vi "XAVIER AUTO.vi"(6 "stop?":bool, 7 "Vision?":bool, 9 "Angle(degrees)":dbl, 10 "Cluster":cluster{"DriveRef":T1}, 11 "Auto Choice":T9(ring)) -> (3 "End?":bool)   [LabVIEW 2015]
uses:
  Robot Global Data.vi
  <vilib>/Rock Robotics/WPI/CAN/Jaguar/SubVIs/WPI_CANJaguar_ControlMode.ctl
  <vilib>/Rock Robotics/WPI/CAN/TalonSRX/WPI_CANTalonSRX_APIControlMode.ctl
  <vilib>/Rock Robotics/SystemInterfaces/DIO/FPGA_DIOPWMChannel.ctl
  <vilib>/Rock Robotics/WPI/PWM/WPI_PWMDeadband.ctl
  <vilib>/Rock Robotics/WPI/MotorControl/WPI_MotorControlType.ctl
  <vilib>/Rock Robotics/WPI/MotorControl/WPI_MotorControlDeviceRef.ctl
  <vilib>/Rock Robotics/WPI/RobotDrive/WPI_RobotDriveDevRef.ctl
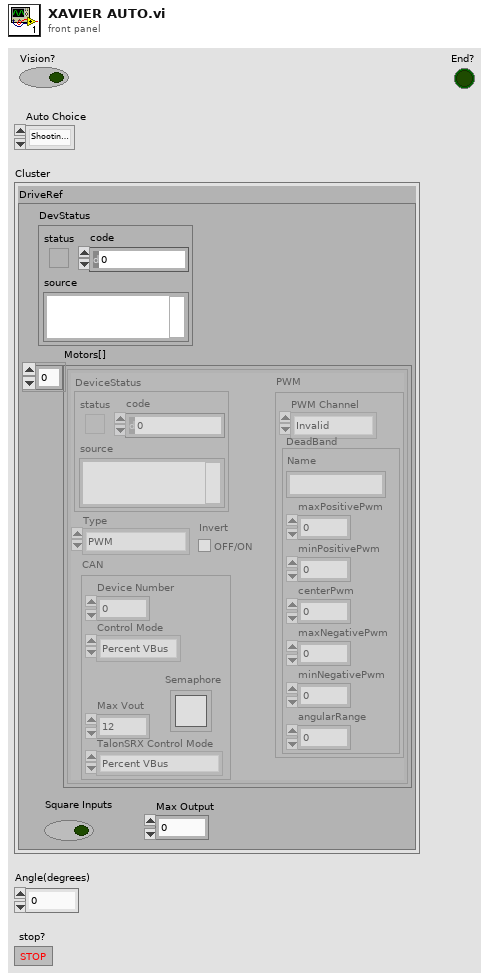
[diagram p1: front panel]
types:
  T1 = typedef "WPI_RobotDriveDevRef.ctl" = cluster{"DevStatus":errorcluster, "Motors[]":T2[], "Square Inputs":bool, "Max Output":dbl}
  T2 = typedef "WPI_MotorControlDeviceRef.ctl" = cluster{"DeviceStatus":errorcluster, "Type":T3, "PWM":cluster{"PWM Channel":T4, "DeadBand":T5}, "CAN":cluster{"Device Number":u8, "Control Mode":T6, "Semaphore":T7, "Max Vout":dbl, "TalonSRX Control Mode":T8}, "Invert":bool}
  T3 = typedef "WPI_MotorControlType.ctl" = enum16{"PWM", "CAN", "CANTalonSRX"}
  T4 = typedef "FPGA_DIOPWMChannel.ctl" = enum8{"PWM 0", "PWM 1", "PWM 2", "PWM 3", "PWM 4", "PWM 5", "PWM 6", "PWM 7", "PWM 8", "PWM 9", "PWM MXP 0", "PWM MXP 1", "PWM MXP 2", "PWM MXP 3", "PWM MXP 4", "PWM MXP 5", "PWM MXP 6", "PWM MXP 7", "PWM MXP 8", "PWM MXP 9", "Invalid"}
  T5 = typedef "WPI_PWMDeadband.ctl" = cluster{"Name":string, "maxPositivePwm":i32, "minPositivePwm":i32, "centerPwm":i32, "maxNegativePwm":i32, "minNegativePwm":i32, "angularRange":u16}
  T6 = typedef "WPI_CANJaguar_ControlMode.ctl" = enum8{"Percent VBus", "Current", "Speed", "Position", "Voltage"}
  T7 = typedef "Semaphore RefNum" = refnum<k1>
  T8 = typedef "WPI_CANTalonSRX_APIControlMode.ctl" = enum8{"Percent VBus", "Speed", "Position", "Slave", "Unchanged / Invalid", "Voltage Compensation", "Current", "Motion Profile"}
  T9 = enum16{"Shooting (Testing Only)", "Low Bar/Pos 2/Pos 3 (full)", "Low Bar/Pos 2/Pos 3 (no turn back)", "Low Bar/Pos 2/Pos 3 (move and turn test)", "Position 4", "Position 5", "Move Arms Down/Up Test", "Move Forward through Defense", "Turn Until Vision Test"}
  T10 = enum16{"Start", "Turn (No Vision)", "Turn (Vision)", "Shoot", "Turn Back", "Move Back", "End"}
  T11 = cluster{"y":dbl, "Distance":dbl, "Angle":dbl, "x":dbl}
  T12 = typedef "WPI_CANTalonSRX_GlobalStatus.ctl" = cluster{"Applied Throttle":dbl, "Module Enabled":bool, "CAN Error":errorcluster, "Closed Loop Error":dbl, "Forward Limit Switch Closed":bool, "Reverse Limit Switch Closed":bool, "Sensor Position":dbl, "Sensor Velocity":dbl, "Current":dbl, "Sticky Fault - Over Temp":bool, "Sticky Fault - Under Voltage":bool, "Sticky Fault - Forward Limit":bool, "Sticky Fault - Reverse Limit":bool, "Sticky Fault - Forward Soft Limit":bool, "Sticky Fault - Reverse Soft Limit":bool, "Brake is Enabled":bool, "Encoder Position":dbl, "Encoder Velocity":dbl, "Encoder Index Count":dbl, "Encoder A Pin State":bool, "Encoder B Pin State":bool, "Encoder Index Pin State":bool, "Analog In":dbl, "Analog In Velocity":dbl, "Temperature (C)":dbl, "Battery Voltage":dbl, "Control 5 Is Supported":bool, "Current Profile Slot Select":dbl, "Pos Div 8":bool, "Vel Div 4":bool, "Pulse Width Position":i32, "Pulse Width Velocity":i32, "Pulse Width Rise To Rise (us)":i32, "Pulse Width Rise To Fall (us)":i32, "Mot Prof Active Is Under Run":bool, "Mot Prof Active Has Under Run":bool, "Mot Prof Active Is Last":bool, "Mot Prof Active Velocity Only":bool, "Mot Prof Active Is Valid":bool, "Mot Prof Buffer Is Full":bool, "Mot Prof Active Profile Slot Select":i32, "Mot Prof NextID":i32, "Mot Prof Count":i32, "Mot Prof Active Velocity":dbl, "Mot Prof Active Position":dbl, "Mot Prof Output Enable":i32}
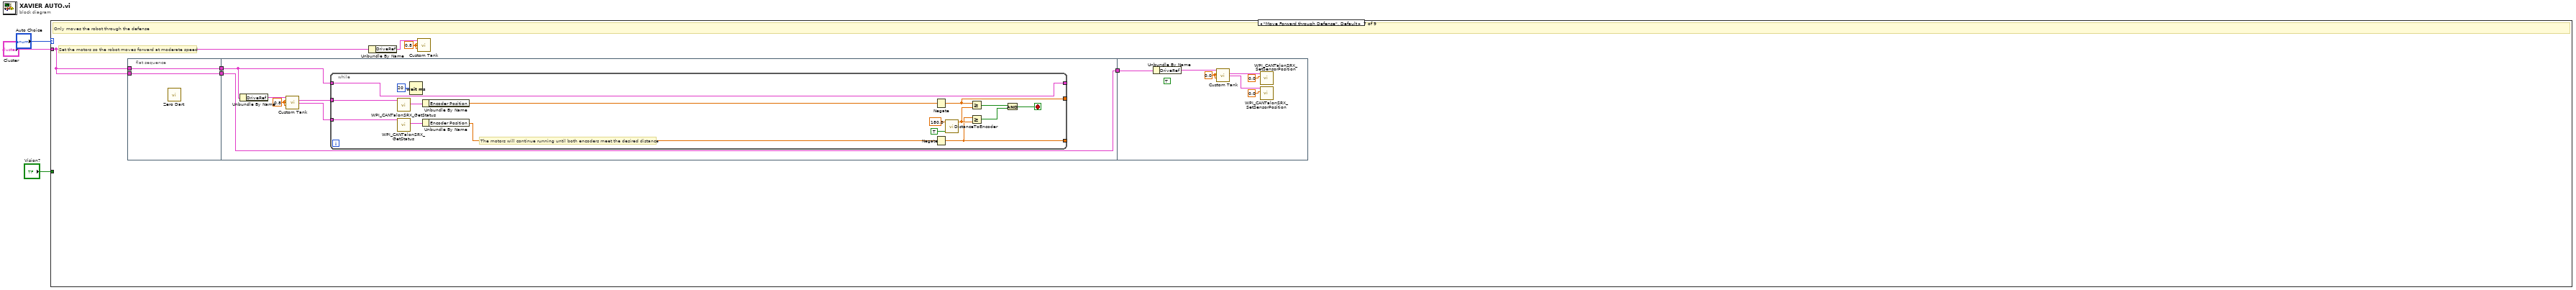
[diagram p0: block diagram]
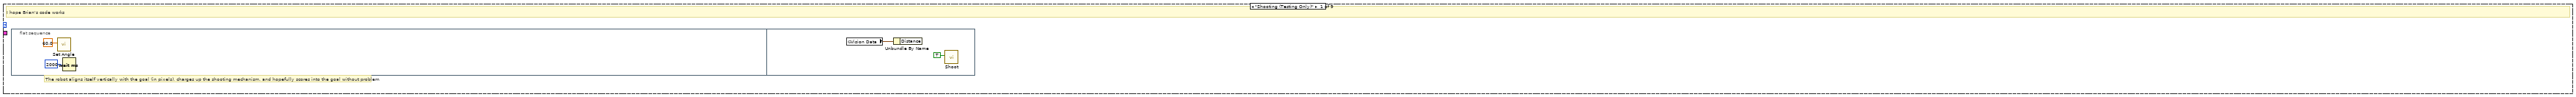
[diagram p2: hidden frame]
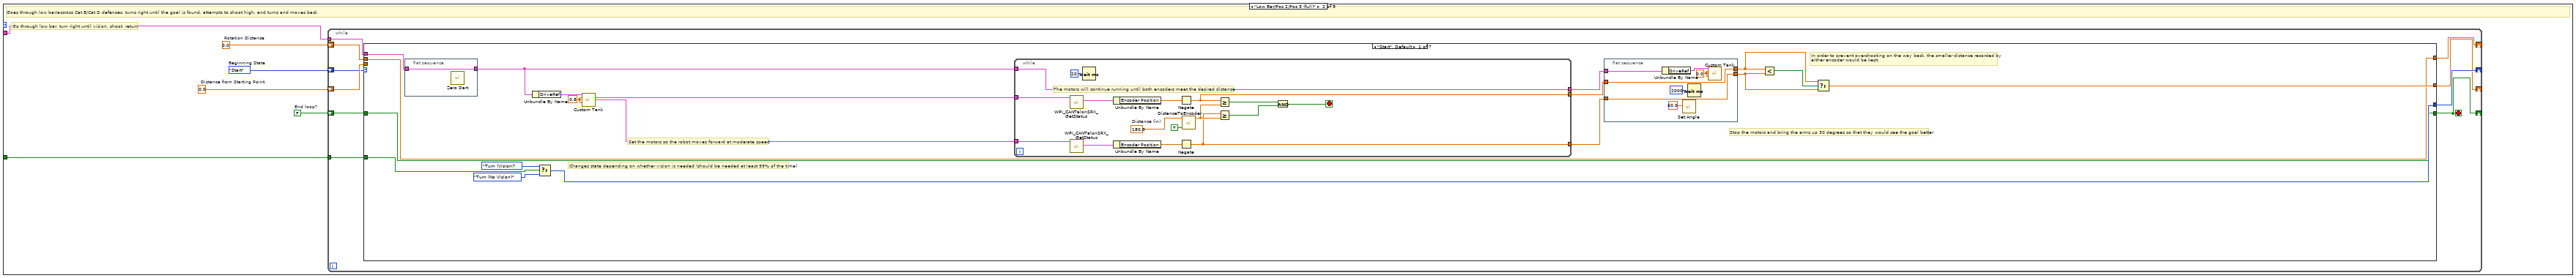
[diagram p3: hidden frame]
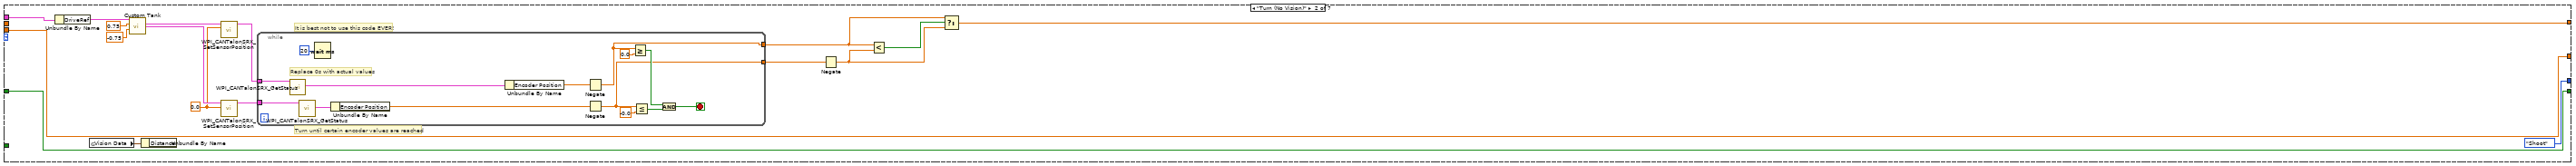
[diagram p4: hidden frame]
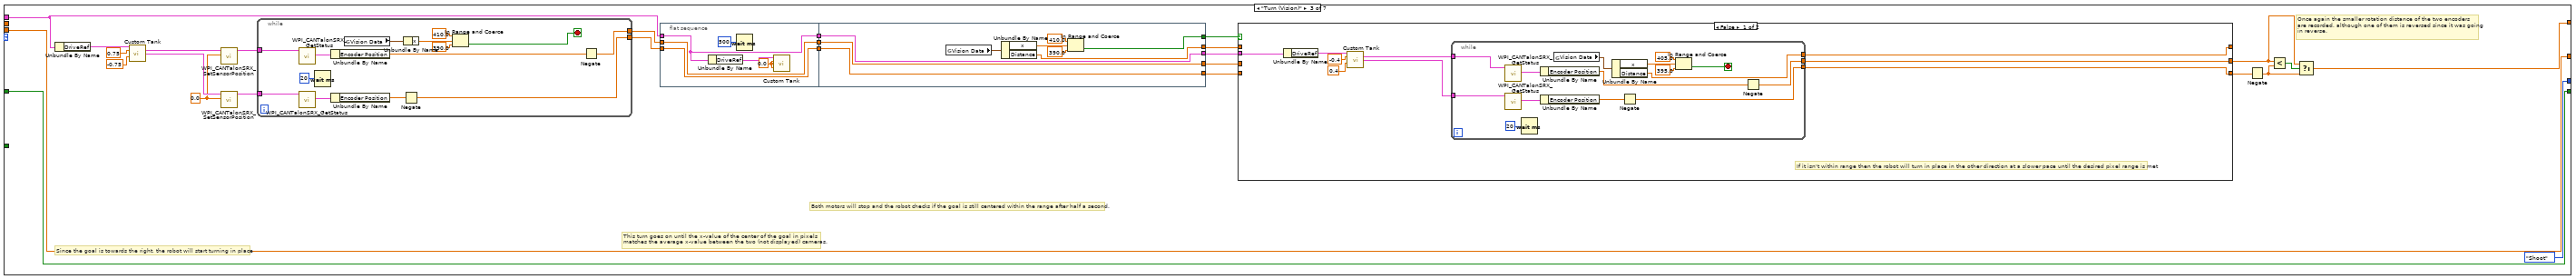
[diagram p5: hidden frame]
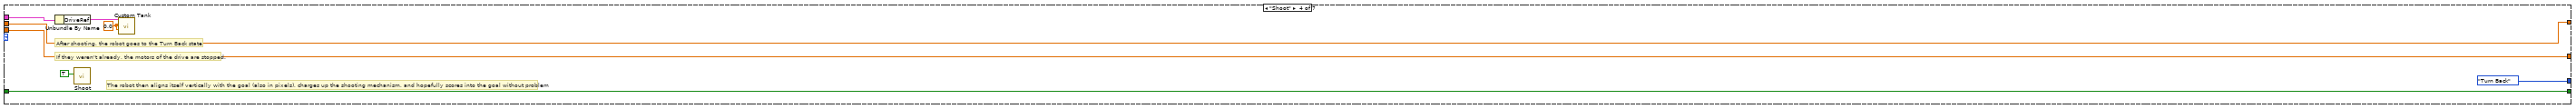
[diagram p7: hidden frame]
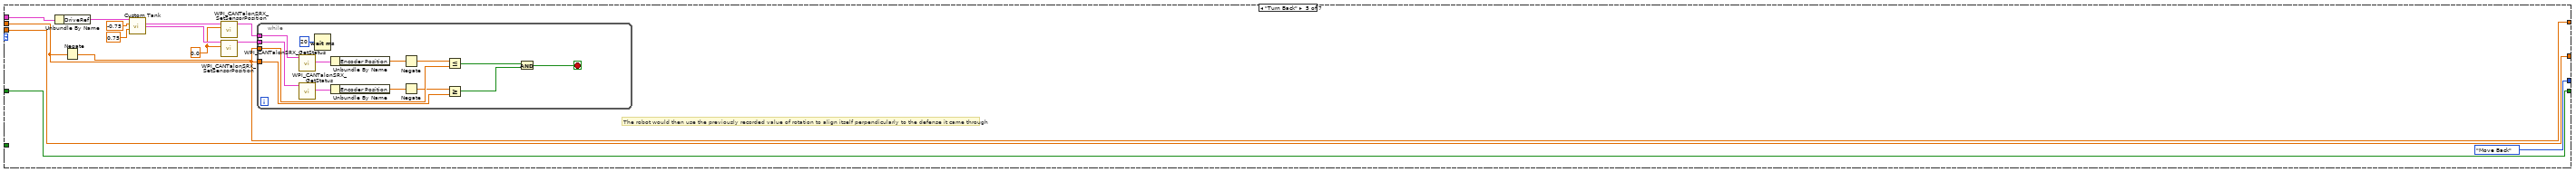
[diagram p8: hidden frame]
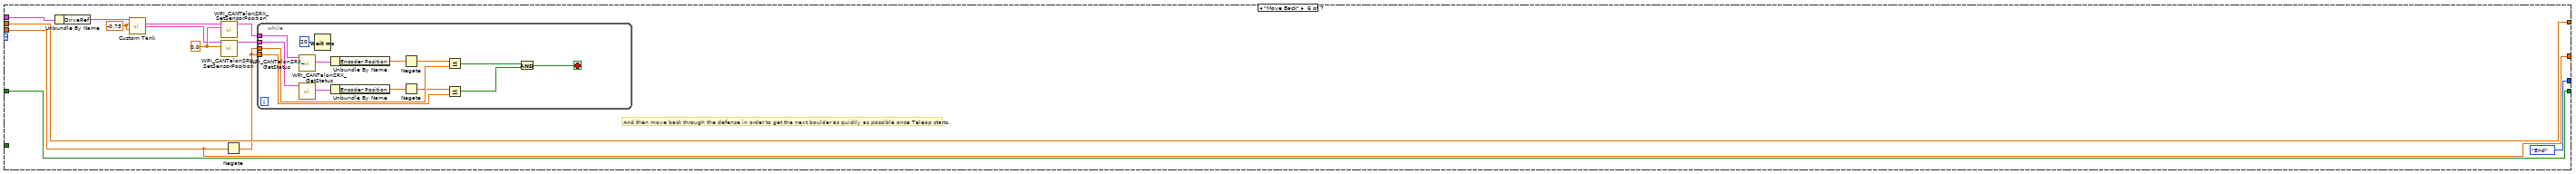
[diagram p9: hidden frame]
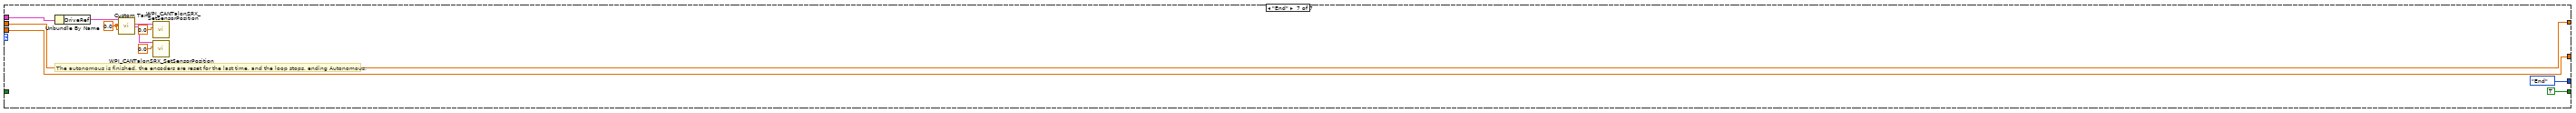
[diagram p10: hidden frame]
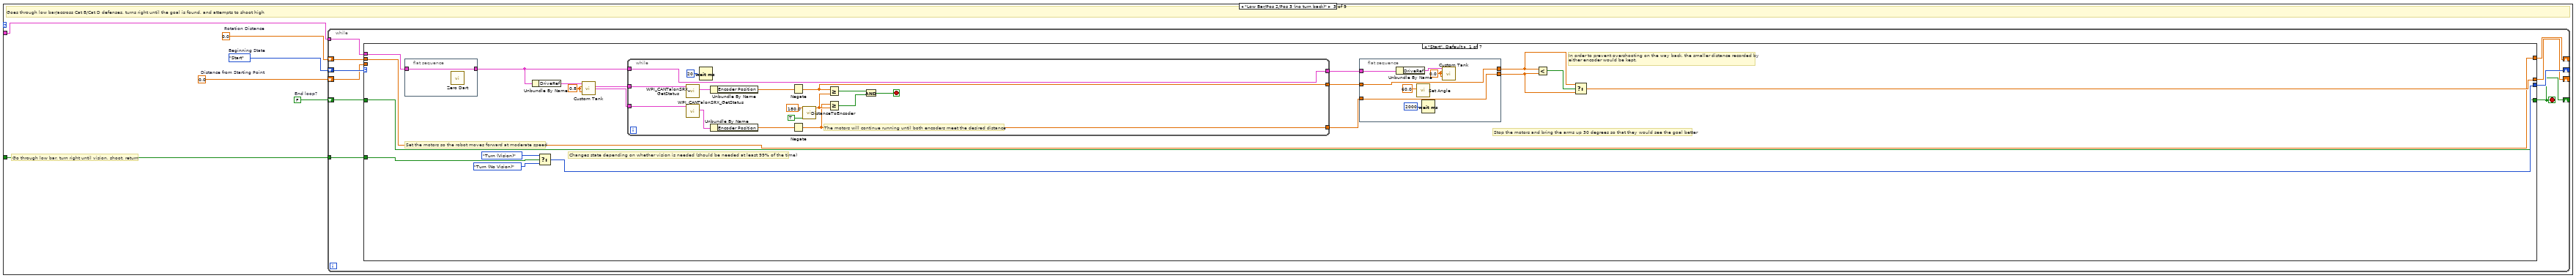
[diagram p11: hidden frame]
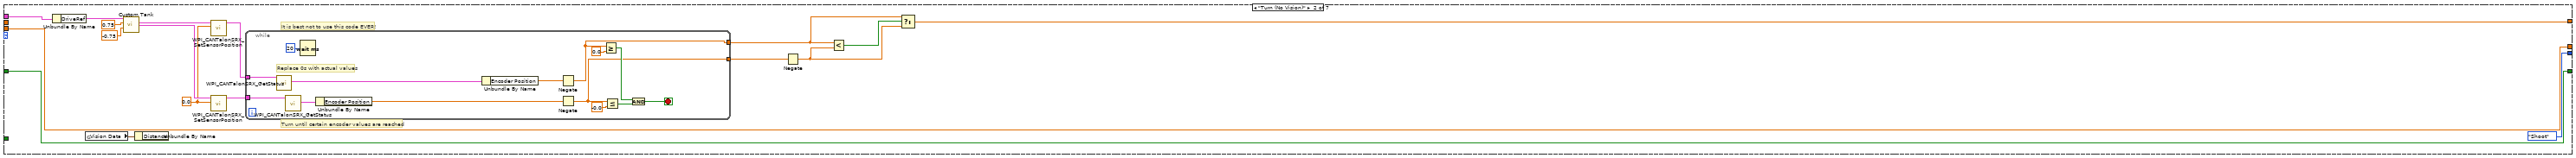
[diagram p12: hidden frame]
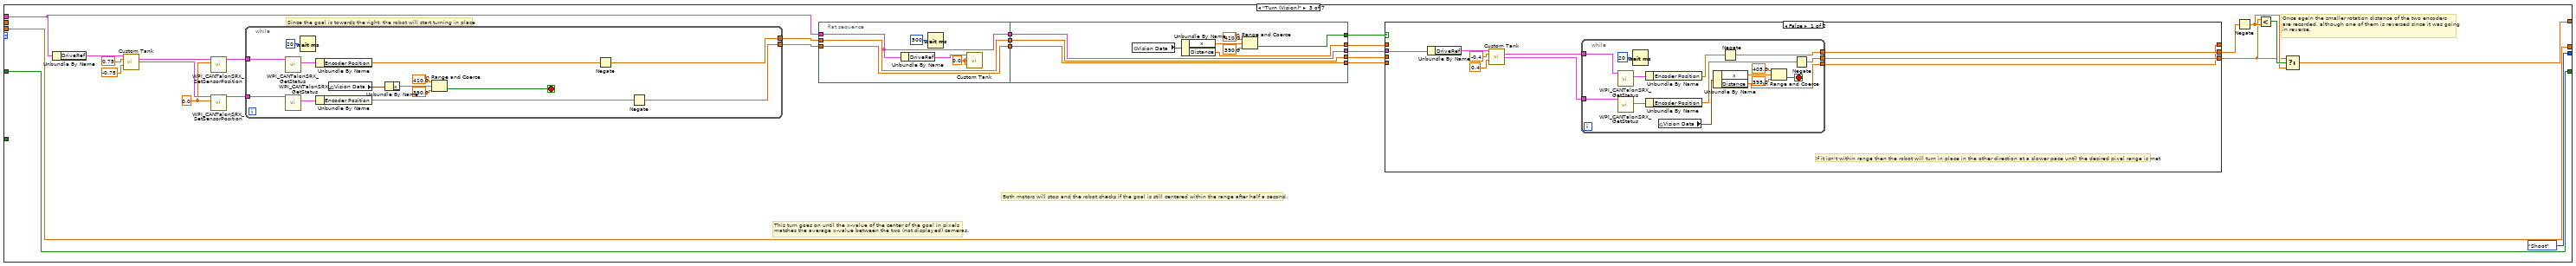
[diagram p13: hidden frame]
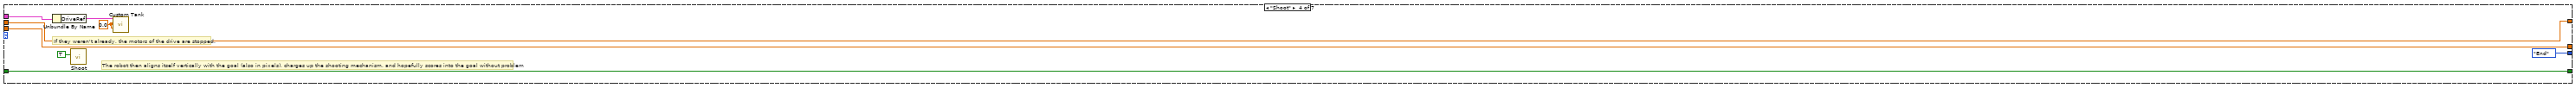
[diagram p15: hidden frame]
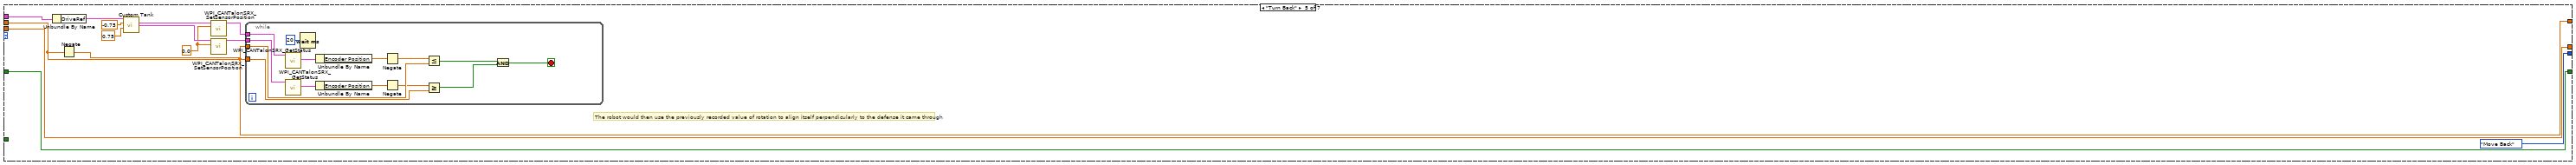
[diagram p16: hidden frame]
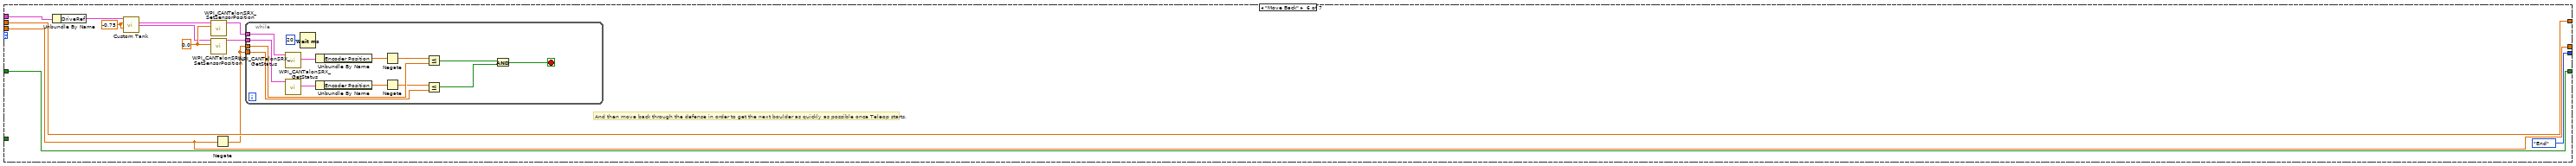
[diagram p17: hidden frame]
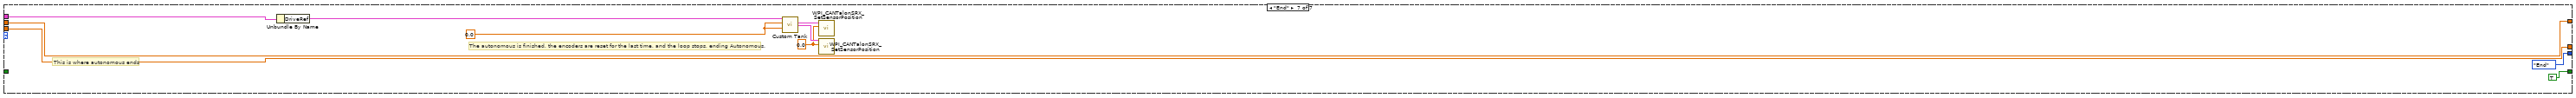
[diagram p18: hidden frame]
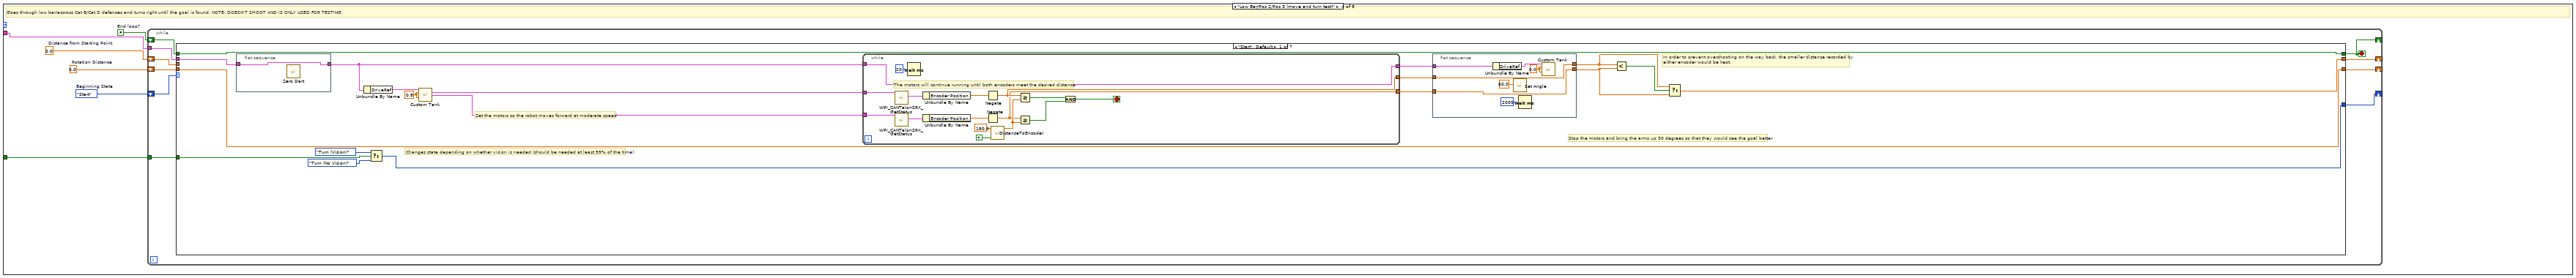
[diagram p19: hidden frame]
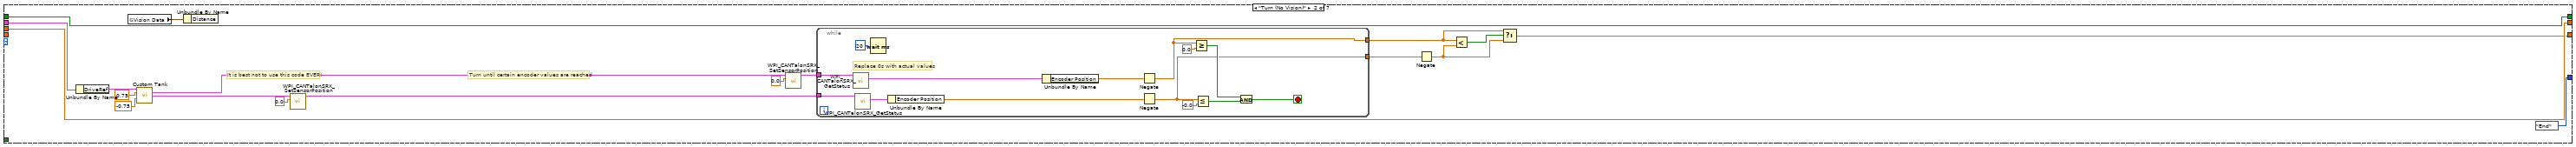
[diagram p20: hidden frame]
diagram:
  n1 = case shown="\"Move Forward through Defense\", Default" "Auto Choice" {
    tunnel: "Vision?" -> [_ w11 w257 w504 _ w859 _ _ _]
    tunnel: "Cluster" -> [_ w8 w256 w503 w755 w858 w1114 w1149 _]
    frame "Shooting (Testing Only)" {
      # "The robot aligns itself vertically with the goal (in pixels), charges up the shooting mechanism, and hopefully scores into the goal without problem"
      # "I hope Brian's code works"
      n2 = flat-sequence {
        frame #0 {
          n3 = call "Set Angle.vi"("Angle(degrees)"=60.0) -> ()  [unwired: 10 in, 1 out]
          n4 = Wait (ms)(milliseconds to wait=u32 2000) -> ()  [unwired: 1 out]
        }
        frame #1 {
          n5 = global read "Robot Global Data.vi" "Vision Data"() -> (w6:T11)
          n6 = Unbundle By Name(w6) -> ()  [unwired: 1 out]
          n7 = call "Shoot.vi"("Trigger"=TRUE ("Aimbot?")) -> ()  [unwired: 8 in, 3 out]
        }
      }
    }
    frame "Low Bar/Pos 2/Pos 3 (full)" {
      w10 = 0.0  # Rotation Distance
      w9 = 0.0  # Distance from Starting Point
      w12 = FALSE  # End loop?
      w13 = T10."Start"  # Beginning State
      # "Go through low bar, turn right until vision, shoot, return"
      # "Goes through low bar/accross Cat B/Cat D defenses, turns right until the goal is found, attempts to shoot high, and turns and moves back"
      n8 = while {
        shift-right: [w23] -> _
        shift-left: w13 -> [w15]
        shift-right: [w21] -> _
        shift-left: w12 -> [w22]
        shift-right: [w19] -> _
        shift-left: w9 -> [w20]
        shift-right: [w17] -> _
        shift-left: w10 -> [w18]
        tunnel: w11 -> [w16]
        tunnel: w8 -> [w14]
        stop <- w21 stop-if-true
        n9 = case shown="\"Start\", Default" w15 {
          tunnel: [w42 T10."Shoot" T10."Shoot" T10."Turn Back" T10."Move Back" T10."End" T10."End"] -> w23
          tunnel: [w41 w83 w121 w189 w202 w229 TRUE] -> w21
          tunnel: w22 -> [w41 w83 w121 w189 w202 w229 _]
          tunnel: [w35 w82 w120 w184 w201 w226 w253] -> w19
          tunnel: w20 -> [_ w82 w120 w184 w201 w226 w253]
          tunnel: w18 -> [w34 _ _ w187 w199 w228 w252]
          tunnel: [w34 w77 w122 w187 w199 w228 w252] -> w17
          tunnel: w16 -> [w33 _ _ _ _ _ _]
          tunnel: w14 -> [w29 w75 w119 w186 w198 w225 w251]
          frame "Start", Default {
            w26 = 0.8 ("LeftMotorsSpeed")
            # "In order to prevent overshooting on the way back, the smaller distance recorded by\neither encoder would be kept."
            # "Stop the motors and bring the arms up 30 degrees so that they would see the goal better"
            # "Set the motors so the robot moves forward at moderate speed"
            # "Changes state depending on whether vision is needed (should be needed at least 99% of the time)"
            n10 = flat-sequence {
              tunnel: w29 -> [w43]
              tunnel: [w43] -> w28
              frame #0 {
                n11 = call "Zero Dart.vi"() -> ()  [unwired: 10 in, 2 out]
              }
            }
            n12 = Unbundle By Name(w28) -> ("DriveRef"=w27:T1)
            n13 = Select(t=T10."Turn (Vision)", s=w33, f=T10."Turn (No Vision)") -> (s? t:f=w42:T10)
            n14 = call "Custom Tank.vi"("RobotDriveDevRef 2"=w27, "Left axis value"=w26, "Right axis value"=w26) -> ("Middle Left Motor"=w25:T2, "Middle Right Motor"=w24:T2)  [unwired: 8 in, 3 out]
            n15 = while {
              tunnel: [w46] -> w31
              tunnel: [w44] -> w30
              tunnel: w28 -> [w52]
              tunnel: [w52] -> w32
              tunnel: w25 -> [w49]
              tunnel: w24 -> [w48]
              stop <- w57 stop-if-true
              w55 = 180.0  # Distance (in)
              # "The motors will continue running until both encoders meet the desired distance"
              n16 = call <vilib>:"WPI_CANTalonSRX_GetStatus.vi"("CAN Talon SRX Ref"=w49) -> ("Talon SRX Status"=w51:T12)  [unwired: 8 in, 2 out]
              n17 = call <vilib>:"WPI_CANTalonSRX_GetStatus.vi"("CAN Talon SRX Ref"=w48) -> ("Talon SRX Status"=w50:T12)  [unwired: 8 in, 2 out]
              n18 = Wait (ms)(milliseconds to wait=u32 20) -> ()  [unwired: 1 out]
              n19 = Unbundle By Name(w51) -> ("Encoder Position"=w47:dbl)
              n20 = Unbundle By Name(w50) -> ("Encoder Position"=w45:dbl)
              n21 = Negate(x=w47) -> (-x=w46:dbl)
              n22 = Negate(x=w45) -> (-x=w44:dbl)
              n23 = call "DistanceToEncoder.vi"(8:TRUE ("Gear Setting"), "Distance (in)"=w55) -> ("Encoder Ticks"=w54:dbl)  [unwired: 9 in]
              n24 = Greater Or Equal?(x=w46, y=w54) -> (x >= y?=w59:bool)
              n25 = Greater Or Equal?(x=w44, y=w54) -> (x >= y?=w58:bool)
              n26 = And(x=w59, y=w58) -> (x .and. y?=w57:bool)
            }
            n27 = flat-sequence {
              tunnel: [w63] -> w37
              tunnel: [w62] -> w36
              tunnel: w32 -> [w64]
              tunnel: w31 -> [w63]
              tunnel: w30 -> [w62]
              frame #0 {
                w60 = 0.0 ("LeftMotorsSpeed")
                n28 = Unbundle By Name(w64) -> ("DriveRef"=w61:T1)
                n29 = call "Set Angle.vi"("Angle(degrees)"=60.0) -> ()  [unwired: 10 in, 1 out]
                n30 = Wait (ms)(milliseconds to wait=u32 2000) -> ()  [unwired: 1 out]
                n31 = call "Custom Tank.vi"("RobotDriveDevRef 2"=w61, "Left axis value"=w60, "Right axis value"=w60) -> ()  [unwired: 8 in, 5 out]
              }
            }
            n32 = Less?(x=w37, y=w36) -> (x < y?=w38:bool)
            n33 = Select(t=w37, s=w38, f=w36) -> (s? t:f=w35:dbl)
          }
          frame "Turn (No Vision)" {
            w67 = 0.0 ("New Sensor Position")
            # "It is best not to use this code EVER!"
            # "Turn until certain encoder values are reached"
            n34 = Unbundle By Name(w75) -> ("DriveRef"=w74:T1)
            n35 = global read "Robot Global Data.vi" "Vision Data"() -> (w76:T11)
            n36 = call "Custom Tank.vi"("RobotDriveDevRef 2"=w74, "Left axis value"=0.75 ("LeftMotorsSpeed"), "Right axis value"=-0.75 ("RightMotorsSpeed")) -> ("Middle Left Motor"=w71:T2, "Middle Right Motor"=w70:T2)  [unwired: 8 in, 3 out]
            n37 = Unbundle By Name(w76) -> ()  [unwired: 1 out]
            n38 = call <vilib>:"WPI_CANTalonSRX_SetSensorPosition.vi"("New Sensor Position"=w67, "CAN Talon SRX Ref"=w71) -> ("CAN Talon SRX Ref"=w69:T2)  [unwired: 8 in, 1 out]
            n39 = call <vilib>:"WPI_CANTalonSRX_SetSensorPosition.vi"("New Sensor Position"=w67, "CAN Talon SRX Ref"=w70) -> ("CAN Talon SRX Ref"=w68:T2)  [unwired: 8 in, 1 out]
            n40 = while {
              tunnel: w69 -> [w91]
              tunnel: w68 -> [w89]
              tunnel: [w87] -> w79
              tunnel: [w85] -> w81
              stop <- w94 stop-if-true
              # "Replace 0s with actual values"
              n41 = call <vilib>:"WPI_CANTalonSRX_GetStatus.vi"("CAN Talon SRX Ref"=w91) -> ("Talon SRX Status"=w92:T12)  [unwired: 8 in, 2 out]
              n42 = call <vilib>:"WPI_CANTalonSRX_GetStatus.vi"("CAN Talon SRX Ref"=w89) -> ("Talon SRX Status"=w90:T12)  [unwired: 8 in, 2 out]
              n43 = Wait (ms)(milliseconds to wait=u32 20) -> ()  [unwired: 1 out]
              n44 = Unbundle By Name(w90) -> ("Encoder Position"=w86:dbl)
              n45 = Unbundle By Name(w92) -> ("Encoder Position"=w88:dbl)
              n46 = Negate(x=w88) -> (-x=w87:dbl)
              n47 = Negate(x=w86) -> (-x=w85:dbl)
              n48 = Greater Or Equal?(x=w87, y=0.0) -> (x >= y?=w97:bool)
              n49 = Less Or Equal?(x=w85, y=-0.0) -> (x <= y?=w96:bool)
              n50 = And(x=w97, y=w96) -> (x .and. y?=w94:bool)
            }
            n51 = Negate(x=w81) -> (-x=w78:dbl)
            n52 = Less?(x=w79, y=w78) -> (x < y?=w80:bool)
            n53 = Select(t=w79, s=w80, f=w78) -> (s? t:f=w77:dbl)
          }
          frame "Turn (Vision)" {
            w99 = 0.0 ("New Sensor Position")
            # "This turn goes on until the x-value of the center of the goal in pixels\nmatches the average x-value between the two (not displayed) cameras."
            # "Once again the smaller rotation distance of the two encoders\nare recorded, although one of them is reversed since it was going\nin reverse."
            # "Both motors will stop and the robot checks if the goal is still centered within the range after half a second."
            # "Since the goal is towards the right, the robot will start turning in place"
            n54 = Unbundle By Name(w119) -> ("DriveRef"=w106:T1)
            n55 = call "Custom Tank.vi"("RobotDriveDevRef 2"=w106, "Left axis value"=0.75 ("LeftMotorsSpeed"), "Right axis value"=-0.75 ("RightMotorsSpeed")) -> ("Middle Left Motor"=w103:T2, "Middle Right Motor"=w102:T2)  [unwired: 8 in, 3 out]
            n56 = call <vilib>:"WPI_CANTalonSRX_SetSensorPosition.vi"("New Sensor Position"=w99, "CAN Talon SRX Ref"=w103) -> ("CAN Talon SRX Ref"=w101:T2)  [unwired: 8 in, 1 out]
            n57 = call <vilib>:"WPI_CANTalonSRX_SetSensorPosition.vi"("New Sensor Position"=w99, "CAN Talon SRX Ref"=w102) -> ("CAN Talon SRX Ref"=w100:T2)  [unwired: 8 in, 1 out]
            n58 = while {
              tunnel: [w153] -> w117
              tunnel: [w155] -> w118
              tunnel: w101 -> [w158]
              tunnel: w100 -> [w157]
              stop <- w162 stop-if-true
              n59 = call <vilib>:"WPI_CANTalonSRX_GetStatus.vi"("CAN Talon SRX Ref"=w158) -> ("Talon SRX Status"=w160:T12)  [unwired: 8 in, 2 out]
              n60 = call <vilib>:"WPI_CANTalonSRX_GetStatus.vi"("CAN Talon SRX Ref"=w157) -> ("Talon SRX Status"=w159:T12)  [unwired: 8 in, 2 out]
              n61 = Wait (ms)(milliseconds to wait=u32 20) -> ()  [unwired: 1 out]
              n62 = Unbundle By Name(w160) -> ("Encoder Position"=w156:dbl)
              n63 = Unbundle By Name(w159) -> ("Encoder Position"=w154:dbl)
              n64 = global read "Robot Global Data.vi" "Vision Data"() -> (w166:T11)
              n65 = Negate(x=w154) -> (-x=w153:dbl)
              n66 = Unbundle By Name(w166) -> ("x"=w165:dbl)
              n67 = In Range and Coerce(upper limit=410.0, x=w165, lower limit=390.0) -> (In Range?=w162:bool)  [unwired: 1 out]
              n68 = Negate(x=w156) -> (-x=w155:dbl)
            }
            n69 = flat-sequence {
              tunnel: w119 -> [w171]
              tunnel: w118 -> [w170]
              tunnel: w117 -> [w169]
              tunnel: [w171] -> w111
              tunnel: [w170] -> w110
              tunnel: [w169] -> w109
              tunnel: [w179] -> w112
              tunnel: [w180] -> w113
              tunnel: [w181] -> w114
              tunnel: w111 -> [w181]
              tunnel: w110 -> [w180]
              tunnel: w109 -> [w179]
              tunnel: [w174] -> w108
              tunnel: [w173] -> w107
              frame #0 {
                w167 = 0.0 ("LeftMotorsSpeed")
                n70 = Unbundle By Name(w171) -> ("DriveRef"=w168:T1)
                n71 = Wait (ms)(milliseconds to wait=u32 500) -> ()  [unwired: 1 out]
                n72 = call "Custom Tank.vi"("RobotDriveDevRef 2"=w168, "Left axis value"=w167, "Right axis value"=w167) -> ()  [unwired: 8 in, 5 out]
              }
              frame #1 {
                n73 = global read "Robot Global Data.vi" "Vision Data"() -> (w178:T11)
                n74 = Unbundle By Name(w178) -> ("x"=w177:dbl, "Distance"=w173:dbl)
                n75 = In Range and Coerce(upper limit=410.0, x=w177, lower limit=390.0) -> (In Range?=w174:bool)  [unwired: 1 out]
              }
            }
            n76 = case shown="False" w108 {
              tunnel: [w133 w152] -> w115
              tunnel: w112 -> [_ w152]
              tunnel: w113 -> [_ w151]
              tunnel: [w134 w151] -> w116
              tunnel: w114 -> [w132 _]
              tunnel: [w131 w150] -> _
              tunnel: w107 -> [_ w150]
              frame False {
                # "If it isn't within range then the robot will turn in place in the other direction at a slower pace until the desired pixel range is met"
                n77 = Unbundle By Name(w132) -> ("DriveRef"=w130:T1)
                n78 = call "Custom Tank.vi"("RobotDriveDevRef 2"=w130, "Left axis value"=-0.4 ("LeftMotorsSpeed"), "Right axis value"=0.4 ("RightMotorsSpeed")) -> ("Middle Left Motor"=w126:T2, "Middle Right Motor"=w127:T2)  [unwired: 8 in, 3 out]
                n79 = while {
                  tunnel: [w137] -> w134
                  tunnel: [w135] -> w133
                  tunnel: [w143] -> w131
                  tunnel: w127 -> [w140]
                  tunnel: w126 -> [w139]
                  stop <- w149 stop-if-true
                  n80 = call <vilib>:"WPI_CANTalonSRX_GetStatus.vi"("CAN Talon SRX Ref"=w139) -> ("Talon SRX Status"=w142:T12)  [unwired: 8 in, 2 out]
                  n81 = call <vilib>:"WPI_CANTalonSRX_GetStatus.vi"("CAN Talon SRX Ref"=w140) -> ("Talon SRX Status"=w141:T12)  [unwired: 8 in, 2 out]
                  n82 = Wait (ms)(milliseconds to wait=u32 20) -> ()  [unwired: 1 out]
                  n83 = Unbundle By Name(w142) -> ("Encoder Position"=w138:dbl)
                  n84 = Unbundle By Name(w141) -> ("Encoder Position"=w136:dbl)
                  n85 = global read "Robot Global Data.vi" "Vision Data"() -> (w148:T11)
                  n86 = Unbundle By Name(w148) -> ("x"=w147:dbl, "Distance"=w143:dbl)
                  n87 = Negate(x=w136) -> (-x=w135:dbl)
                  n88 = In Range and Coerce(upper limit=405.0, x=w147, lower limit=395.0) -> (In Range?=w149:bool)  [unwired: 1 out]
                  n89 = Negate(x=w138) -> (-x=w137:dbl)
                }
              }
              frame True {
                # "If it is within range, then the robot moves on to the shooting state"
              }
            }
            n90 = Negate(x=w115) -> (-x=w124:dbl)
            n91 = Less?(x=w116, y=w124) -> (x < y?=w125:bool)
            n92 = Select(t=w116, s=w125, f=w124) -> (s? t:f=w122:dbl)
          }
          frame "Shoot" {
            w182 = 0.0 ("LeftMotorsSpeed")
            # "After shooting, the robot goes to the Turn Back state"
            # "If they weren't already, the motors of the drive are stopped."
            # "The robot then aligns itself vertically with the goal (also in pixels), charges up the shooting mechanism, and hopefully scores into the goal without problem"
            n93 = Unbundle By Name(w186) -> ("DriveRef"=w183:T1)
            n94 = call "Shoot.vi"("Trigger"=TRUE ("Collection Trigger")) -> ()  [unwired: 8 in, 3 out]
            n95 = call "Custom Tank.vi"("RobotDriveDevRef 2"=w183, "Left axis value"=w182, "Right axis value"=w182) -> ()  [unwired: 8 in, 5 out]
          }
          frame "Turn Back" {
            w190 = 0.0 ("New Sensor Position")
            # "The robot would then use the previously recorded value of rotation to align itself perpendicularly to the defense it came through"
            n96 = Unbundle By Name(w198) -> ("DriveRef"=w197:T1)
            n97 = Negate(x=w199) -> (-x=w200:dbl)
            n98 = call "Custom Tank.vi"("RobotDriveDevRef 2"=w197, "Left axis value"=-0.75 ("LeftMotorsSpeed"), "Right axis value"=0.75 ("RightMotorsSpeed")) -> ("Middle Left Motor"=w191:T2, "Middle Right Motor"=w192:T2)  [unwired: 8 in, 3 out]
            n99 = call <vilib>:"WPI_CANTalonSRX_SetSensorPosition.vi"("New Sensor Position"=w190, "CAN Talon SRX Ref"=w191) -> ("CAN Talon SRX Ref"=w194:T2)  [unwired: 8 in, 1 out]
            n100 = call <vilib>:"WPI_CANTalonSRX_SetSensorPosition.vi"("New Sensor Position"=w190, "CAN Talon SRX Ref"=w192) -> ("CAN Talon SRX Ref"=w193:T2)  [unwired: 8 in, 1 out]
            n101 = while {
              tunnel: w194 -> [w209]
              tunnel: w193 -> [w208]
              tunnel: w199 -> [w214]
              tunnel: w200 -> [w213]
              stop <- w215 stop-if-true
              n102 = call <vilib>:"WPI_CANTalonSRX_GetStatus.vi"("CAN Talon SRX Ref"=w209) -> ("Talon SRX Status"=w211:T12)  [unwired: 8 in, 2 out]
              n103 = call <vilib>:"WPI_CANTalonSRX_GetStatus.vi"("CAN Talon SRX Ref"=w208) -> ("Talon SRX Status"=w210:T12)  [unwired: 8 in, 2 out]
              n104 = Wait (ms)(milliseconds to wait=u32 20) -> ()  [unwired: 1 out]
              n105 = Unbundle By Name(w211) -> ("Encoder Position"=w207:dbl)
              n106 = Unbundle By Name(w210) -> ("Encoder Position"=w204:dbl)
              n107 = Negate(x=w207) -> (-x=w206:dbl)
              n108 = Negate(x=w204) -> (-x=w205:dbl)
              n109 = Less Or Equal?(x=w206, y=w213) -> (x <= y?=w217:bool)
              n110 = Greater Or Equal?(x=w205, y=w214) -> (x >= y?=w216:bool)
              n111 = And(x=w217, y=w216) -> (x .and. y?=w215:bool)
            }
          }
          frame "Move Back" {
            w222 = 0.0 ("New Sensor Position")
            w223 = -0.75 ("LeftMotorsSpeed")
            # "And then move back through the defense in order to get the next boulder as quickly as possible once Teleop starts."
            n112 = Unbundle By Name(w225) -> ("DriveRef"=w224:T1)
            n113 = call "Custom Tank.vi"("RobotDriveDevRef 2"=w224, "Left axis value"=w223, "Right axis value"=w223) -> ("Middle Left Motor"=w221:T2, "Middle Right Motor"=w220:T2)  [unwired: 8 in, 3 out]
            n114 = call <vilib>:"WPI_CANTalonSRX_SetSensorPosition.vi"("New Sensor Position"=w222, "CAN Talon SRX Ref"=w221) -> ("CAN Talon SRX Ref"=w219:T2)  [unwired: 8 in, 1 out]
            n115 = call <vilib>:"WPI_CANTalonSRX_SetSensorPosition.vi"("New Sensor Position"=w222, "CAN Talon SRX Ref"=w220) -> ("CAN Talon SRX Ref"=w218:T2)  [unwired: 8 in, 1 out]
            n116 = Negate(x=w226) -> (-x=w227:dbl)
            n117 = while {
              tunnel: w219 -> [w237]
              tunnel: w218 -> [w235]
              tunnel: w227 -> [w241]
              tunnel: w227 -> [w240]
              stop <- w242 stop-if-true
              n118 = call <vilib>:"WPI_CANTalonSRX_GetStatus.vi"("CAN Talon SRX Ref"=w237) -> ("Talon SRX Status"=w238:T12)  [unwired: 8 in, 2 out]
              n119 = call <vilib>:"WPI_CANTalonSRX_GetStatus.vi"("CAN Talon SRX Ref"=w235) -> ("Talon SRX Status"=w236:T12)  [unwired: 8 in, 2 out]
              n120 = Wait (ms)(milliseconds to wait=u32 20) -> ()  [unwired: 1 out]
              n121 = Unbundle By Name(w238) -> ("Encoder Position"=w234:dbl)
              n122 = Unbundle By Name(w236) -> ("Encoder Position"=w232:dbl)
              n123 = Negate(x=w234) -> (-x=w233:dbl)
              n124 = Negate(x=w232) -> (-x=w231:dbl)
              n125 = Less Or Equal?(x=w233, y=w241) -> (x <= y?=w244:bool)
              n126 = Less Or Equal?(x=w231, y=w240) -> (x <= y?=w243:bool)
              n127 = And(x=w244, y=w243) -> (x .and. y?=w242:bool)
            }
          }
          frame "End" {
            w249 = 0.0 ("Left axis value")
            # "The autonomous is finished, the encoders are reset for the last time, and the loop stops, ending Autonomous."
            n128 = Unbundle By Name(w251) -> ("DriveRef"=w250:T1)
            n129 = call "Custom Tank.vi"("RobotDriveDevRef 2"=w250, "Left axis value"=w249, "Right axis value"=w249) -> ("Middle Left Motor"=w246:T2, "Middle Right Motor"=w245:T2)  [unwired: 8 in, 3 out]
            n130 = call <vilib>:"WPI_CANTalonSRX_SetSensorPosition.vi"("New Sensor Position"=0.0, "CAN Talon SRX Ref"=w246) -> ()  [unwired: 8 in, 2 out]
            n131 = call <vilib>:"WPI_CANTalonSRX_SetSensorPosition.vi"("New Sensor Position"=0.0, "CAN Talon SRX Ref"=w245) -> ()  [unwired: 8 in, 2 out]
          }
        }
      }
    }
    frame "Low Bar/Pos 2/Pos 3 (no turn back)" {
      w258 = 0.0  # Rotation Distance
      w259 = 0.0  # Distance from Starting Point
      w260 = FALSE  # End loop?
      w261 = T10."Start"  # Beginning State
      # "Go through low bar, turn right until vision, shoot, return"
      # "Goes through low bar/accross Cat B/Cat D defenses, turns right until the goal is found, and attempts to shoot high"
      n132 = while {
        shift-right: [w270] -> _
        shift-left: w261 -> [w271]
        shift-right: [w268] -> _
        shift-left: w260 -> [w269]
        shift-right: [w266] -> _
        shift-left: w259 -> [w267]
        shift-right: [w264] -> _
        shift-left: w258 -> [w265]
        tunnel: w257 -> [w263]
        tunnel: w256 -> [w262]
        stop <- w268 stop-if-true
        n133 = case shown="\"Start\", Default" w271 {
          tunnel: [w290 T10."Shoot" T10."Shoot" T10."End" T10."Move Back" T10."End" T10."End"] -> w270
          tunnel: [w289 w331 w369 w437 w446 w477 TRUE] -> w268
          tunnel: w269 -> [w289 w331 w369 w437 w446 w477 _]
          tunnel: [w283 w330 w368 w435 w450 w474 w500] -> w266
          tunnel: w267 -> [_ w330 w368 w435 w450 w474 w500]
          tunnel: w265 -> [w282 _ _ w434 w448 w476 w499]
          tunnel: [w282 w325 w370 w434 w448 w476 w499] -> w264
          tunnel: w263 -> [w281 _ _ _ _ _ _]
          tunnel: w262 -> [w274 w323 w365 w433 w447 w473 w498]
          frame "Start", Default {
            w276 = 0.8 ("LeftMotorsSpeed")
            # "In order to prevent overshooting on the way back, the smaller distance recorded by\neither encoder would be kept."
            # "Stop the motors and bring the arms up 30 degrees so that they would see the goal better"
            # "Set the motors so the robot moves forward at moderate speed"
            # "Changes state depending on whether vision is needed (should be needed at least 99% of the time)"
            n134 = flat-sequence {
              tunnel: w274 -> [w291]
              tunnel: [w291] -> w275
              frame #0 {
                n135 = call "Zero Dart.vi"() -> ()  [unwired: 10 in, 2 out]
              }
            }
            n136 = Unbundle By Name(w275) -> ("DriveRef"=w277:T1)
            n137 = Select(t=T10."Turn (Vision)", s=w281, f=T10."Turn (No Vision)") -> (s? t:f=w290:T10)
            n138 = call "Custom Tank.vi"("RobotDriveDevRef 2"=w277, "Left axis value"=w276, "Right axis value"=w276) -> ("Middle Left Motor"=w273:T2, "Middle Right Motor"=w272:T2)  [unwired: 8 in, 3 out]
            n139 = while {
              tunnel: [w294] -> w279
              tunnel: [w293] -> w278
              tunnel: w275 -> [w300]
              tunnel: [w300] -> w280
              tunnel: w273 -> [w297]
              tunnel: w272 -> [w296]
              stop <- w305 stop-if-true
              # "The motors will continue running until both encoders meet the desired distance"
              n140 = call <vilib>:"WPI_CANTalonSRX_GetStatus.vi"("CAN Talon SRX Ref"=w297) -> ("Talon SRX Status"=w299:T12)  [unwired: 8 in, 2 out]
              n141 = call <vilib>:"WPI_CANTalonSRX_GetStatus.vi"("CAN Talon SRX Ref"=w296) -> ("Talon SRX Status"=w298:T12)  [unwired: 8 in, 2 out]
              n142 = Wait (ms)(milliseconds to wait=u32 20) -> ()  [unwired: 1 out]
              n143 = Unbundle By Name(w299) -> ("Encoder Position"=w295:dbl)
              n144 = Unbundle By Name(w298) -> ("Encoder Position"=w292:dbl)
              n145 = Negate(x=w295) -> (-x=w294:dbl)
              n146 = Negate(x=w292) -> (-x=w293:dbl)
              n147 = call "DistanceToEncoder.vi"(8:TRUE ("Gear Setting"), "Distance (in)"=180.0 ("Distance")) -> ("Encoder Ticks"=w303:dbl)  [unwired: 9 in]
              n148 = Greater Or Equal?(x=w294, y=w303) -> (x >= y?=w307:bool)
              n149 = Greater Or Equal?(x=w293, y=w303) -> (x >= y?=w306:bool)
              n150 = And(x=w307, y=w306) -> (x .and. y?=w305:bool)
            }
            n151 = flat-sequence {
              tunnel: [w311] -> w285
              tunnel: [w310] -> w284
              tunnel: w280 -> [w312]
              tunnel: w279 -> [w311]
              tunnel: w278 -> [w310]
              frame #0 {
                w308 = 0.0 ("LeftMotorsSpeed")
                n152 = Unbundle By Name(w312) -> ("DriveRef"=w309:T1)
                n153 = call "Set Angle.vi"("Angle(degrees)"=60.0) -> ()  [unwired: 10 in, 1 out]
                n154 = Wait (ms)(milliseconds to wait=u32 2000) -> ()  [unwired: 1 out]
                n155 = call "Custom Tank.vi"("RobotDriveDevRef 2"=w309, "Left axis value"=w308, "Right axis value"=w308) -> ()  [unwired: 8 in, 5 out]
              }
            }
            n156 = Less?(x=w285, y=w284) -> (x < y?=w286:bool)
            n157 = Select(t=w285, s=w286, f=w284) -> (s? t:f=w283:dbl)
          }
          frame "Turn (No Vision)" {
            w317 = 0.0 ("New Sensor Position")
            # "It is best not to use this code EVER!"
            # "Turn until certain encoder values are reached"
            n158 = Unbundle By Name(w323) -> ("DriveRef"=w322:T1)
            n159 = global read "Robot Global Data.vi" "Vision Data"() -> (w324:T11)
            n160 = call "Custom Tank.vi"("RobotDriveDevRef 2"=w322, "Left axis value"=0.75 ("LeftMotorsSpeed"), "Right axis value"=-0.75 ("RightMotorsSpeed")) -> ("Middle Left Motor"=w319:T2, "Middle Right Motor"=w318:T2)  [unwired: 8 in, 3 out]
            n161 = Unbundle By Name(w324) -> ()  [unwired: 1 out]
            n162 = call <vilib>:"WPI_CANTalonSRX_SetSensorPosition.vi"("New Sensor Position"=w317, "CAN Talon SRX Ref"=w319) -> ("CAN Talon SRX Ref"=w316:T2)  [unwired: 8 in, 1 out]
            n163 = call <vilib>:"WPI_CANTalonSRX_SetSensorPosition.vi"("New Sensor Position"=w317, "CAN Talon SRX Ref"=w318) -> ("CAN Talon SRX Ref"=w315:T2)  [unwired: 8 in, 1 out]
            n164 = while {
              tunnel: w316 -> [w341]
              tunnel: w315 -> [w339]
              tunnel: [w333] -> w327
              tunnel: [w335] -> w329
              stop <- w343 stop-if-true
              # "Replace 0s with actual values"
              n165 = call <vilib>:"WPI_CANTalonSRX_GetStatus.vi"("CAN Talon SRX Ref"=w341) -> ("Talon SRX Status"=w340:T12)  [unwired: 8 in, 2 out]
              n166 = call <vilib>:"WPI_CANTalonSRX_GetStatus.vi"("CAN Talon SRX Ref"=w339) -> ("Talon SRX Status"=w338:T12)  [unwired: 8 in, 2 out]
              n167 = Wait (ms)(milliseconds to wait=u32 20) -> ()  [unwired: 1 out]
              n168 = Unbundle By Name(w338) -> ("Encoder Position"=w337:dbl)
              n169 = Unbundle By Name(w340) -> ("Encoder Position"=w334:dbl)
              n170 = Negate(x=w334) -> (-x=w333:dbl)
              n171 = Negate(x=w337) -> (-x=w335:dbl)
              n172 = Greater Or Equal?(x=w333, y=0.0) -> (x >= y?=w345:bool)
              n173 = Less Or Equal?(x=w335, y=-0.0) -> (x <= y?=w336:bool)
              n174 = And(x=w345, y=w336) -> (x .and. y?=w343:bool)
            }
            n175 = Negate(x=w329) -> (-x=w326:dbl)
            n176 = Less?(x=w327, y=w326) -> (x < y?=w328:bool)
            n177 = Select(t=w327, s=w328, f=w326) -> (s? t:f=w325:dbl)
          }
          frame "Turn (Vision)" {
            w349 = 0.0 ("New Sensor Position")
            # "This turn goes on until the x-value of the center of the goal in pixels\nmatches the average x-value between the two (not displayed) cameras."
            # "Once again the smaller rotation distance of the two encoders\nare recorded, although one of them is reversed since it was going\nin reverse."
            # "Both motors will stop and the robot checks if the goal is still centered within the range after half a second."
            # "Since the goal is towards the right, the robot will start turning in place"
            n178 = Unbundle By Name(w365) -> ("DriveRef"=w354:T1)
            n179 = call "Custom Tank.vi"("RobotDriveDevRef 2"=w354, "Left axis value"=0.75 ("LeftMotorsSpeed"), "Right axis value"=-0.75 ("RightMotorsSpeed")) -> ("Middle Left Motor"=w351:T2, "Middle Right Motor"=w350:T2)  [unwired: 8 in, 3 out]
            n180 = call <vilib>:"WPI_CANTalonSRX_SetSensorPosition.vi"("New Sensor Position"=w349, "CAN Talon SRX Ref"=w351) -> ("CAN Talon SRX Ref"=w348:T2)  [unwired: 8 in, 1 out]
            n181 = call <vilib>:"WPI_CANTalonSRX_SetSensorPosition.vi"("New Sensor Position"=w349, "CAN Talon SRX Ref"=w350) -> ("CAN Talon SRX Ref"=w347:T2)  [unwired: 8 in, 1 out]
            n182 = while {
              tunnel: w348 -> [w407]
              tunnel: w347 -> [w405]
              tunnel: [w403] -> w367
              tunnel: [w401] -> w366
              stop <- w410 stop-if-true
              n183 = call <vilib>:"WPI_CANTalonSRX_GetStatus.vi"("CAN Talon SRX Ref"=w407) -> ("Talon SRX Status"=w408:T12)  [unwired: 8 in, 2 out]
              n184 = call <vilib>:"WPI_CANTalonSRX_GetStatus.vi"("CAN Talon SRX Ref"=w405) -> ("Talon SRX Status"=w406:T12)  [unwired: 8 in, 2 out]
              n185 = Wait (ms)(milliseconds to wait=u32 20) -> ()  [unwired: 1 out]
              n186 = Unbundle By Name(w408) -> ("Encoder Position"=w404:dbl)
              n187 = Unbundle By Name(w406) -> ("Encoder Position"=w402:dbl)
              n188 = global read "Robot Global Data.vi" "Vision Data"() -> (w414:T11)
              n189 = Unbundle By Name(w414) -> ("x"=w413:dbl)
              n190 = In Range and Coerce(upper limit=410.0, x=w413, lower limit=390.0) -> (In Range?=w410:bool)  [unwired: 1 out]
              n191 = Negate(x=w404) -> (-x=w403:dbl)
              n192 = Negate(x=w402) -> (-x=w401:dbl)
            }
            n193 = flat-sequence {
              tunnel: w367 -> [w417]
              tunnel: w366 -> [w418]
              tunnel: w365 -> [w419]
              tunnel: [w419] -> w359
              tunnel: [w418] -> w358
              tunnel: [w417] -> w357
              tunnel: [w427] -> w362
              tunnel: [w428] -> w363
              tunnel: [w429] -> w364
              tunnel: w359 -> [w429]
              tunnel: w358 -> [w428]
              tunnel: w357 -> [w427]
              tunnel: [w422] -> w356
              tunnel: [w421] -> w355
              frame #0 {
                w416 = 0.0 ("LeftMotorsSpeed")
                n194 = Unbundle By Name(w419) -> ("DriveRef"=w415:T1)
                n195 = Wait (ms)(milliseconds to wait=u32 500) -> ()  [unwired: 1 out]
                n196 = call "Custom Tank.vi"("RobotDriveDevRef 2"=w415, "Left axis value"=w416, "Right axis value"=w416) -> ()  [unwired: 8 in, 5 out]
              }
              frame #1 {
                n197 = global read "Robot Global Data.vi" "Vision Data"() -> (w426:T11)
                n198 = Unbundle By Name(w426) -> ("x"=w425:dbl, "Distance"=w421:dbl)
                n199 = In Range and Coerce(upper limit=410.0, x=w425, lower limit=390.0) -> (In Range?=w422:bool)  [unwired: 1 out]
              }
            }
            n200 = case shown="False" w356 {
              tunnel: [w381 w400] -> w361
              tunnel: w362 -> [_ w400]
              tunnel: w363 -> [_ w399]
              tunnel: [w382 w399] -> w360
              tunnel: w364 -> [w380 _]
              tunnel: [w379 w398] -> _
              tunnel: w355 -> [_ w398]
              frame False {
                # "If it isn't within range then the robot will turn in place in the other direction at a slower pace until the desired pixel range is met"
                n201 = Unbundle By Name(w380) -> ("DriveRef"=w378:T1)
                n202 = call "Custom Tank.vi"("RobotDriveDevRef 2"=w378, "Left axis value"=-0.4 ("LeftMotorsSpeed"), "Right axis value"=0.4 ("RightMotorsSpeed")) -> ("Middle Left Motor"=w375:T2, "Middle Right Motor"=w374:T2)  [unwired: 8 in, 3 out]
                n203 = while {
                  tunnel: [w384] -> w382
                  tunnel: [w385] -> w381
                  tunnel: [w391] -> w379
                  tunnel: w375 -> [w388]
                  tunnel: w374 -> [w387]
                  stop <- w397 stop-if-true
                  n204 = call <vilib>:"WPI_CANTalonSRX_GetStatus.vi"("CAN Talon SRX Ref"=w388) -> ("Talon SRX Status"=w390:T12)  [unwired: 8 in, 2 out]
                  n205 = call <vilib>:"WPI_CANTalonSRX_GetStatus.vi"("CAN Talon SRX Ref"=w387) -> ("Talon SRX Status"=w389:T12)  [unwired: 8 in, 2 out]
                  n206 = Wait (ms)(milliseconds to wait=u32 20) -> ()  [unwired: 1 out]
                  n207 = Unbundle By Name(w390) -> ("Encoder Position"=w386:dbl)
                  n208 = Unbundle By Name(w389) -> ("Encoder Position"=w383:dbl)
                  n209 = global read "Robot Global Data.vi" "Vision Data"() -> (w396:T11)
                  n210 = Unbundle By Name(w396) -> ("x"=w395:dbl, "Distance"=w391:dbl)
                  n211 = Negate(x=w386) -> (-x=w385:dbl)
                  n212 = In Range and Coerce(upper limit=405.0, x=w395, lower limit=395.0) -> (In Range?=w397:bool)  [unwired: 1 out]
                  n213 = Negate(x=w383) -> (-x=w384:dbl)
                }
              }
              frame True {
                # "If it is within range, then the robot moves on to the shooting state"
              }
            }
            n214 = Negate(x=w361) -> (-x=w372:dbl)
            n215 = Less?(x=w360, y=w372) -> (x < y?=w373:bool)
            n216 = Select(t=w360, s=w373, f=w372) -> (s? t:f=w370:dbl)
          }
          frame "Shoot" {
            w430 = 0.0 ("LeftMotorsSpeed")
            # "If they weren't already, the motors of the drive are stopped."
            # "The robot then aligns itself vertically with the goal (also in pixels), charges up the shooting mechanism, and hopefully scores into the goal without problem"
            n217 = Unbundle By Name(w433) -> ("DriveRef"=w431:T1)
            n218 = call "Shoot.vi"("Trigger"=TRUE ("Collection Trigger")) -> ()  [unwired: 8 in, 3 out]
            n219 = call "Custom Tank.vi"("RobotDriveDevRef 2"=w431, "Left axis value"=w430, "Right axis value"=w430) -> ()  [unwired: 8 in, 5 out]
          }
          frame "Turn Back" {
            w440 = 0.0 ("New Sensor Position")
            # "The robot would then use the previously recorded value of rotation to align itself perpendicularly to the defense it came through"
            n220 = Unbundle By Name(w447) -> ("DriveRef"=w445:T1)
            n221 = Negate(x=w448) -> (-x=w449:dbl)
            n222 = call "Custom Tank.vi"("RobotDriveDevRef 2"=w445, "Left axis value"=-0.75 ("LeftMotorsSpeed"), "Right axis value"=0.75 ("RightMotorsSpeed")) -> ("Middle Left Motor"=w442:T2, "Middle Right Motor"=w441:T2)  [unwired: 8 in, 3 out]
            n223 = call <vilib>:"WPI_CANTalonSRX_SetSensorPosition.vi"("New Sensor Position"=w440, "CAN Talon SRX Ref"=w442) -> ("CAN Talon SRX Ref"=w439:T2)  [unwired: 8 in, 1 out]
            n224 = call <vilib>:"WPI_CANTalonSRX_SetSensorPosition.vi"("New Sensor Position"=w440, "CAN Talon SRX Ref"=w441) -> ("CAN Talon SRX Ref"=w438:T2)  [unwired: 8 in, 1 out]
            n225 = while {
              tunnel: w439 -> [w458]
              tunnel: w438 -> [w456]
              tunnel: w448 -> [w462]
              tunnel: w449 -> [w461]
              stop <- w463 stop-if-true
              n226 = call <vilib>:"WPI_CANTalonSRX_GetStatus.vi"("CAN Talon SRX Ref"=w458) -> ("Talon SRX Status"=w459:T12)  [unwired: 8 in, 2 out]
              n227 = call <vilib>:"WPI_CANTalonSRX_GetStatus.vi"("CAN Talon SRX Ref"=w456) -> ("Talon SRX Status"=w457:T12)  [unwired: 8 in, 2 out]
              n228 = Wait (ms)(milliseconds to wait=u32 20) -> ()  [unwired: 1 out]
              n229 = Unbundle By Name(w459) -> ("Encoder Position"=w455:dbl)
              n230 = Unbundle By Name(w457) -> ("Encoder Position"=w453:dbl)
              n231 = Negate(x=w455) -> (-x=w454:dbl)
              n232 = Negate(x=w453) -> (-x=w452:dbl)
              n233 = Less Or Equal?(x=w454, y=w461) -> (x <= y?=w465:bool)
              n234 = Greater Or Equal?(x=w452, y=w462) -> (x >= y?=w464:bool)
              n235 = And(x=w465, y=w464) -> (x .and. y?=w463:bool)
            }
          }
          frame "Move Back" {
            w470 = 0.0 ("New Sensor Position")
            w471 = -0.75 ("LeftMotorsSpeed")
            # "And then move back through the defense in order to get the next boulder as quickly as possible once Teleop starts."
            n236 = Unbundle By Name(w473) -> ("DriveRef"=w472:T1)
            n237 = call "Custom Tank.vi"("RobotDriveDevRef 2"=w472, "Left axis value"=w471, "Right axis value"=w471) -> ("Middle Left Motor"=w469:T2, "Middle Right Motor"=w468:T2)  [unwired: 8 in, 3 out]
            n238 = call <vilib>:"WPI_CANTalonSRX_SetSensorPosition.vi"("New Sensor Position"=w470, "CAN Talon SRX Ref"=w469) -> ("CAN Talon SRX Ref"=w467:T2)  [unwired: 8 in, 1 out]
            n239 = call <vilib>:"WPI_CANTalonSRX_SetSensorPosition.vi"("New Sensor Position"=w470, "CAN Talon SRX Ref"=w468) -> ("CAN Talon SRX Ref"=w466:T2)  [unwired: 8 in, 1 out]
            n240 = Negate(x=w474) -> (-x=w475:dbl)
            n241 = while {
              tunnel: w467 -> [w486]
              tunnel: w466 -> [w484]
              tunnel: w475 -> [w490]
              tunnel: w475 -> [w489]
              stop <- w491 stop-if-true
              n242 = call <vilib>:"WPI_CANTalonSRX_GetStatus.vi"("CAN Talon SRX Ref"=w486) -> ("Talon SRX Status"=w487:T12)  [unwired: 8 in, 2 out]
              n243 = call <vilib>:"WPI_CANTalonSRX_GetStatus.vi"("CAN Talon SRX Ref"=w484) -> ("Talon SRX Status"=w485:T12)  [unwired: 8 in, 2 out]
              n244 = Wait (ms)(milliseconds to wait=u32 20) -> ()  [unwired: 1 out]
              n245 = Unbundle By Name(w487) -> ("Encoder Position"=w482:dbl)
              n246 = Unbundle By Name(w485) -> ("Encoder Position"=w479:dbl)
              n247 = Negate(x=w482) -> (-x=w481:dbl)
              n248 = Negate(x=w479) -> (-x=w480:dbl)
              n249 = Less Or Equal?(x=w481, y=w490) -> (x <= y?=w483:bool)
              n250 = Less Or Equal?(x=w480, y=w489) -> (x <= y?=w492:bool)
              n251 = And(x=w483, y=w492) -> (x .and. y?=w491:bool)
            }
          }
          frame "End" {
            w493 = 0.0 ("New Sensor Position")
            w496 = 0.0 ("Left axis value")
            # "The autonomous is finished, the encoders are reset for the last time, and the loop stops, ending Autonomous."
            # "This is where autonomous ends"
            n252 = Unbundle By Name(w498) -> ("DriveRef"=w497:T1)
            n253 = call "Custom Tank.vi"("RobotDriveDevRef 2"=w497, "Left axis value"=w496, "Right axis value"=w496) -> ("Middle Left Motor"=w495:T2, "Middle Right Motor"=w494:T2)  [unwired: 8 in, 3 out]
            n254 = call <vilib>:"WPI_CANTalonSRX_SetSensorPosition.vi"("New Sensor Position"=w493, "CAN Talon SRX Ref"=w495) -> ()  [unwired: 8 in, 2 out]
            n255 = call <vilib>:"WPI_CANTalonSRX_SetSensorPosition.vi"("New Sensor Position"=w493, "CAN Talon SRX Ref"=w494) -> ()  [unwired: 8 in, 2 out]
          }
        }
      }
    }
    frame "Low Bar/Pos 2/Pos 3 (move and turn test)" {
      w505 = 0.0  # Rotation Distance
      w506 = 0.0  # Distance from Starting Point
      w507 = FALSE  # End loop?
      w508 = T10."Start"  # Beginning State
      # "Goes through low bar/accross Cat B/Cat D defenses,and turns right until the goal is found. NOTE: DOESN'T SHOOT AND IS ONLY USED FOR TESTING."
      n256 = while {
        shift-right: [w517] -> _
        shift-left: w508 -> [w518]
        shift-right: [w515] -> _
        shift-left: w507 -> [w516]
        shift-right: [w513] -> _
        shift-left: w506 -> [w514]
        shift-right: [w511] -> _
        shift-left: w505 -> [w512]
        tunnel: w504 -> [w510]
        tunnel: w503 -> [w509]
        stop <- w515 stop-if-true
        n257 = case shown="\"Start\", Default" w518 {
          tunnel: [w537 T10."End" T10."End" T10."Turn Back" T10."Move Back" T10."End" T10."End"] -> w517
          tunnel: [w536 w579 w621 w686 w700 w728 TRUE] -> w515
          tunnel: w516 -> [w536 w579 w621 w686 w700 w728 _]
          tunnel: [w530 w578 w620 w684 w699 w725 w752] -> w513
          tunnel: w514 -> [_ w578 w620 w684 w699 w725 w752]
          tunnel: w512 -> [w529 _ _ w683 w697 w727 w751]
          tunnel: [w529 w573 w617 w683 w697 w727 w751] -> w511
          tunnel: w510 -> [w528 _ _ _ _ _ _]
          tunnel: w509 -> [w522 w571 w614 w682 w696 w724 w750]
          frame "Start", Default {
            w523 = 0.8 ("LeftMotorsSpeed")
            # "In order to prevent overshooting on the way back, the smaller distance recorded by\neither encoder would be kept."
            # "Stop the motors and bring the arms up 30 degrees so that they would see the goal better"
            # "Set the motors so the robot moves forward at moderate speed"
            # "Changes state depending on whether vision is needed (should be needed at least 99% of the time)"
            n258 = flat-sequence {
              tunnel: w522 -> [w538]
              tunnel: [w538] -> w521
              frame #0 {
                n259 = call "Zero Dart.vi"() -> ()  [unwired: 10 in, 2 out]
              }
            }
            n260 = Unbundle By Name(w521) -> ("DriveRef"=w524:T1)
            n261 = Select(t=T10."Turn (Vision)", s=w528, f=T10."Turn (No Vision)") -> (s? t:f=w537:T10)
            n262 = call "Custom Tank.vi"("RobotDriveDevRef 2"=w524, "Left axis value"=w523, "Right axis value"=w523) -> ("Middle Left Motor"=w520:T2, "Middle Right Motor"=w519:T2)  [unwired: 8 in, 3 out]
            n263 = while {
              tunnel: [w542] -> w526
              tunnel: [w539] -> w525
              tunnel: w521 -> [w547]
              tunnel: [w547] -> w527
              tunnel: w520 -> [w544]
              tunnel: w519 -> [w543]
              stop <- w552 stop-if-true
              # "The motors will continue running until both encoders meet the desired distance"
              n264 = call <vilib>:"WPI_CANTalonSRX_GetStatus.vi"("CAN Talon SRX Ref"=w544) -> ("Talon SRX Status"=w546:T12)  [unwired: 8 in, 2 out]
              n265 = call <vilib>:"WPI_CANTalonSRX_GetStatus.vi"("CAN Talon SRX Ref"=w543) -> ("Talon SRX Status"=w545:T12)  [unwired: 8 in, 2 out]
              n266 = Wait (ms)(milliseconds to wait=u32 20) -> ()  [unwired: 1 out]
              n267 = Unbundle By Name(w546) -> ("Encoder Position"=w541:dbl)
              n268 = Unbundle By Name(w545) -> ("Encoder Position"=w540:dbl)
              n269 = Negate(x=w541) -> (-x=w542:dbl)
              n270 = Negate(x=w540) -> (-x=w539:dbl)
              n271 = call "DistanceToEncoder.vi"(8:TRUE ("Gear Setting"), "Distance (in)"=180.0 ("Distance")) -> ("Encoder Ticks"=w549:dbl)  [unwired: 9 in]
              n272 = Greater Or Equal?(x=w542, y=w549) -> (x >= y?=w554:bool)
              n273 = Greater Or Equal?(x=w539, y=w549) -> (x >= y?=w553:bool)
              n274 = And(x=w554, y=w553) -> (x .and. y?=w552:bool)
            }
            n275 = flat-sequence {
              tunnel: [w558] -> w532
              tunnel: [w557] -> w531
              tunnel: w527 -> [w559]
              tunnel: w526 -> [w558]
              tunnel: w525 -> [w557]
              frame #0 {
                w555 = 0.0 ("LeftMotorsSpeed")
                n276 = Unbundle By Name(w559) -> ("DriveRef"=w556:T1)
                n277 = call "Set Angle.vi"("Angle(degrees)"=60.0) -> ()  [unwired: 10 in, 1 out]
                n278 = Wait (ms)(milliseconds to wait=u32 2000) -> ()  [unwired: 1 out]
                n279 = call "Custom Tank.vi"("RobotDriveDevRef 2"=w556, "Left axis value"=w555, "Right axis value"=w555) -> ()  [unwired: 8 in, 5 out]
              }
            }
            n280 = Less?(x=w532, y=w531) -> (x < y?=w533:bool)
            n281 = Select(t=w532, s=w533, f=w531) -> (s? t:f=w530:dbl)
          }
          frame "Turn (No Vision)" {
            # "It is best not to use this code EVER!"
            # "Turn until certain encoder values are reached"
            n282 = Unbundle By Name(w571) -> ("DriveRef"=w570:T1)
            n283 = global read "Robot Global Data.vi" "Vision Data"() -> (w572:T11)
            n284 = call "Custom Tank.vi"("RobotDriveDevRef 2"=w570, "Left axis value"=0.75 ("LeftMotorsSpeed"), "Right axis value"=-0.75 ("RightMotorsSpeed")) -> ("Middle Left Motor"=w563:T2, "Middle Right Motor"=w562:T2)  [unwired: 8 in, 3 out]
            n285 = Unbundle By Name(w572) -> ()  [unwired: 1 out]
            n286 = call <vilib>:"WPI_CANTalonSRX_SetSensorPosition.vi"("New Sensor Position"=0.0, "CAN Talon SRX Ref"=w562) -> ("CAN Talon SRX Ref"=w565:T2)  [unwired: 8 in, 1 out]
            n287 = call <vilib>:"WPI_CANTalonSRX_SetSensorPosition.vi"("New Sensor Position"=0.0, "CAN Talon SRX Ref"=w563) -> ("CAN Talon SRX Ref"=w564:T2)  [unwired: 8 in, 1 out]
            n288 = while {
              tunnel: w564 -> [w586]
              tunnel: w565 -> [w585]
              tunnel: [w583] -> w575
              tunnel: [w581] -> w577
              stop <- w590 stop-if-true
              # "Replace 0s with actual values"
              n289 = call <vilib>:"WPI_CANTalonSRX_GetStatus.vi"("CAN Talon SRX Ref"=w586) -> ("Talon SRX Status"=w588:T12)  [unwired: 8 in, 2 out]
              n290 = call <vilib>:"WPI_CANTalonSRX_GetStatus.vi"("CAN Talon SRX Ref"=w585) -> ("Talon SRX Status"=w587:T12)  [unwired: 8 in, 2 out]
              n291 = Wait (ms)(milliseconds to wait=u32 20) -> ()  [unwired: 1 out]
              n292 = Unbundle By Name(w587) -> ("Encoder Position"=w582:dbl)
              n293 = Unbundle By Name(w588) -> ("Encoder Position"=w584:dbl)
              n294 = Negate(x=w584) -> (-x=w583:dbl)
              n295 = Negate(x=w582) -> (-x=w581:dbl)
              n296 = Greater Or Equal?(x=w583, y=0.0) -> (x >= y?=w593:bool)
              n297 = Less Or Equal?(x=w581, y=-0.0) -> (x <= y?=w592:bool)
              n298 = And(x=w593, y=w592) -> (x .and. y?=w590:bool)
            }
            n299 = Negate(x=w577) -> (-x=w574:dbl)
            n300 = Less?(x=w575, y=w574) -> (x < y?=w576:bool)
            n301 = Select(t=w575, s=w576, f=w574) -> (s? t:f=w573:dbl)
          }
          frame "Turn (Vision)" {
            # "This turn goes on until the x-value of the center of the goal in pixels\nmatches the average x-value between the two (not displayed) cameras."
            # "Once again the smaller rotation distance of the two encoders\nare recorded, although one of them is reversed since it was going\nin reverse."
            # "Since the goal is towards the right, the robot will start turning in place"
            # "Both motors will stop and the robot checks if the goal is still centered within the range after half a second."
            n302 = Unbundle By Name(w614) -> ("DriveRef"=w603:T1)
            n303 = call "Custom Tank.vi"("RobotDriveDevRef 2"=w603, "Left axis value"=0.75 ("LeftMotorsSpeed"), "Right axis value"=-0.75 ("RightMotorsSpeed")) -> ("Middle Left Motor"=w596:T2, "Middle Right Motor"=w595:T2)  [unwired: 8 in, 3 out]
            n304 = call <vilib>:"WPI_CANTalonSRX_SetSensorPosition.vi"("New Sensor Position"=0.0, "CAN Talon SRX Ref"=w596) -> ("CAN Talon SRX Ref"=w598:T2)  [unwired: 8 in, 1 out]
            n305 = call <vilib>:"WPI_CANTalonSRX_SetSensorPosition.vi"("New Sensor Position"=0.0, "CAN Talon SRX Ref"=w595) -> ("CAN Talon SRX Ref"=w597:T2)  [unwired: 8 in, 1 out]
            n306 = while {
              tunnel: w597 -> [w654]
              tunnel: w598 -> [w655]
              tunnel: [w650] -> w615
              tunnel: [w652] -> w616
              stop <- w659 stop-if-true
              n307 = call <vilib>:"WPI_CANTalonSRX_GetStatus.vi"("CAN Talon SRX Ref"=w655) -> ("Talon SRX Status"=w657:T12)  [unwired: 8 in, 2 out]
              n308 = call <vilib>:"WPI_CANTalonSRX_GetStatus.vi"("CAN Talon SRX Ref"=w654) -> ("Talon SRX Status"=w656:T12)  [unwired: 8 in, 2 out]
              n309 = Wait (ms)(milliseconds to wait=u32 20) -> ()  [unwired: 1 out]
              n310 = Unbundle By Name(w657) -> ("Encoder Position"=w653:dbl)
              n311 = Unbundle By Name(w656) -> ("Encoder Position"=w651:dbl)
              n312 = global read "Robot Global Data.vi" "Vision Data"() -> (w663:T11)
              n313 = Unbundle By Name(w663) -> ("x"=w662:dbl)
              n314 = Negate(x=w651) -> (-x=w650:dbl)
              n315 = In Range and Coerce(upper limit=410.0, x=w662, lower limit=390.0) -> (In Range?=w659:bool)  [unwired: 1 out]
              n316 = Negate(x=w653) -> (-x=w652:dbl)
            }
            n317 = flat-sequence {
              tunnel: w616 -> [w667]
              tunnel: w615 -> [w666]
              tunnel: w614 -> [w668]
              tunnel: [w668] -> w608
              tunnel: [w667] -> w607
              tunnel: [w666] -> w606
              tunnel: [w676] -> w611
              tunnel: [w677] -> w612
              tunnel: [w678] -> w613
              tunnel: w608 -> [w678]
              tunnel: w607 -> [w677]
              tunnel: w606 -> [w676]
              tunnel: [w671] -> w605
              tunnel: [w670] -> w604
              frame #0 {
                w664 = 0.0 ("LeftMotorsSpeed")
                n318 = Unbundle By Name(w668) -> ("DriveRef"=w665:T1)
                n319 = Wait (ms)(milliseconds to wait=u32 500) -> ()  [unwired: 1 out]
                n320 = call "Custom Tank.vi"("RobotDriveDevRef 2"=w665, "Left axis value"=w664, "Right axis value"=w664) -> ()  [unwired: 8 in, 5 out]
              }
              frame #1 {
                n321 = global read "Robot Global Data.vi" "Vision Data"() -> (w675:T11)
                n322 = Unbundle By Name(w675) -> ("x"=w674:dbl, "Distance"=w670:dbl)
                n323 = In Range and Coerce(upper limit=410.0, x=w674, lower limit=390.0) -> (In Range?=w671:bool)  [unwired: 1 out]
              }
            }
            n324 = case shown="False" w605 {
              tunnel: [w630 w649] -> w609
              tunnel: w611 -> [_ w649]
              tunnel: w612 -> [_ w648]
              tunnel: [w631 w648] -> w610
              tunnel: w613 -> [w629 _]
              tunnel: [w628 w647] -> _
              tunnel: w604 -> [_ w647]
              frame False {
                # "If it isn't within range then the robot will turn in place in the other direction at a slower pace until the desired pixel range is met"
                n325 = Unbundle By Name(w629) -> ("DriveRef"=w627:T1)
                n326 = call "Custom Tank.vi"("RobotDriveDevRef 2"=w627, "Left axis value"=-0.4 ("LeftMotorsSpeed"), "Right axis value"=0.4 ("RightMotorsSpeed")) -> ("Middle Left Motor"=w624:T2, "Middle Right Motor"=w623:T2)  [unwired: 8 in, 3 out]
                n327 = while {
                  tunnel: [w634] -> w631
                  tunnel: [w632] -> w630
                  tunnel: [w640] -> w628
                  tunnel: w624 -> [w638]
                  tunnel: w623 -> [w636]
                  stop <- w646 stop-if-true
                  n328 = call <vilib>:"WPI_CANTalonSRX_GetStatus.vi"("CAN Talon SRX Ref"=w638) -> ("Talon SRX Status"=w639:T12)  [unwired: 8 in, 2 out]
                  n329 = call <vilib>:"WPI_CANTalonSRX_GetStatus.vi"("CAN Talon SRX Ref"=w636) -> ("Talon SRX Status"=w637:T12)  [unwired: 8 in, 2 out]
                  n330 = Wait (ms)(milliseconds to wait=u32 20) -> ()  [unwired: 1 out]
                  n331 = Unbundle By Name(w639) -> ("Encoder Position"=w635:dbl)
                  n332 = Unbundle By Name(w637) -> ("Encoder Position"=w633:dbl)
                  n333 = global read "Robot Global Data.vi" "Vision Data"() -> (w645:T11)
                  n334 = Unbundle By Name(w645) -> ("x"=w644:dbl, "Distance"=w640:dbl)
                  n335 = Negate(x=w633) -> (-x=w632:dbl)
                  n336 = In Range and Coerce(upper limit=405.0, x=w644, lower limit=395.0) -> (In Range?=w646:bool)  [unwired: 1 out]
                  n337 = Negate(x=w635) -> (-x=w634:dbl)
                }
              }
              frame True {
                # "If it is within range, then the robot moves on to the shooting state"
              }
            }
            n338 = Negate(x=w609) -> (-x=w618:dbl)
            n339 = Less?(x=w610, y=w618) -> (x < y?=w619:bool)
            n340 = Select(t=w610, s=w619, f=w618) -> (s? t:f=w617:dbl)
          }
          frame "Shoot" {
            w679 = 0.0 ("LeftMotorsSpeed")
            # "If they weren't already, the motors of the drive are stopped."
            # "The robot then aligns itself vertically with the goal (also in pixels), charges up the shooting mechanism, and hopefully scores into the goal without problem"
            n341 = Unbundle By Name(w682) -> ("DriveRef"=w680:T1)
            n342 = call "Shoot.vi"("Trigger"=TRUE ("Collection Trigger")) -> ()  [unwired: 8 in, 3 out]
            n343 = call "Custom Tank.vi"("RobotDriveDevRef 2"=w680, "Left axis value"=w679, "Right axis value"=w679) -> ()  [unwired: 8 in, 5 out]
          }
          frame "Turn Back" {
            # "The robot would then use the previously recorded value of rotation to align itself perpendicularly to the defense it came through"
            n344 = Unbundle By Name(w696) -> ("DriveRef"=w695:T1)
            n345 = Negate(x=w697) -> (-x=w698:dbl)
            n346 = call "Custom Tank.vi"("RobotDriveDevRef 2"=w695, "Left axis value"=-0.75 ("LeftMotorsSpeed"), "Right axis value"=0.75 ("RightMotorsSpeed")) -> ("Middle Left Motor"=w688:T2, "Middle Right Motor"=w687:T2)  [unwired: 8 in, 3 out]
            n347 = call <vilib>:"WPI_CANTalonSRX_SetSensorPosition.vi"("New Sensor Position"=0.0, "CAN Talon SRX Ref"=w688) -> ("CAN Talon SRX Ref"=w689:T2)  [unwired: 8 in, 1 out]
            n348 = call <vilib>:"WPI_CANTalonSRX_SetSensorPosition.vi"("New Sensor Position"=0.0, "CAN Talon SRX Ref"=w687) -> ("CAN Talon SRX Ref"=w690:T2)  [unwired: 8 in, 1 out]
            n349 = while {
              tunnel: w689 -> [w707]
              tunnel: w690 -> [w706]
              tunnel: w697 -> [w712]
              tunnel: w698 -> [w711]
              stop <- w713 stop-if-true
              n350 = call <vilib>:"WPI_CANTalonSRX_GetStatus.vi"("CAN Talon SRX Ref"=w707) -> ("Talon SRX Status"=w709:T12)  [unwired: 8 in, 2 out]
              n351 = call <vilib>:"WPI_CANTalonSRX_GetStatus.vi"("CAN Talon SRX Ref"=w706) -> ("Talon SRX Status"=w708:T12)  [unwired: 8 in, 2 out]
              n352 = Wait (ms)(milliseconds to wait=u32 20) -> ()  [unwired: 1 out]
              n353 = Unbundle By Name(w709) -> ("Encoder Position"=w704:dbl)
              n354 = Unbundle By Name(w708) -> ("Encoder Position"=w702:dbl)
              n355 = Negate(x=w704) -> (-x=w705:dbl)
              n356 = Negate(x=w702) -> (-x=w703:dbl)
              n357 = Less Or Equal?(x=w705, y=w711) -> (x <= y?=w715:bool)
              n358 = Greater Or Equal?(x=w703, y=w712) -> (x >= y?=w714:bool)
              n359 = And(x=w715, y=w714) -> (x .and. y?=w713:bool)
            }
          }
          frame "Move Back" {
            w722 = -0.75 ("LeftMotorsSpeed")
            # "And then move back through the defense in order to get the next boulder as quickly as possible once Teleop starts."
            n360 = Unbundle By Name(w724) -> ("DriveRef"=w723:T1)
            n361 = call "Custom Tank.vi"("RobotDriveDevRef 2"=w723, "Left axis value"=w722, "Right axis value"=w722) -> ("Middle Left Motor"=w717:T2, "Middle Right Motor"=w716:T2)  [unwired: 8 in, 3 out]
            n362 = Negate(x=w725) -> (-x=w726:dbl)
            n363 = call <vilib>:"WPI_CANTalonSRX_SetSensorPosition.vi"("New Sensor Position"=0.0, "CAN Talon SRX Ref"=w717) -> ("CAN Talon SRX Ref"=w718:T2)  [unwired: 8 in, 1 out]
            n364 = call <vilib>:"WPI_CANTalonSRX_SetSensorPosition.vi"("New Sensor Position"=0.0, "CAN Talon SRX Ref"=w716) -> ("CAN Talon SRX Ref"=w719:T2)  [unwired: 8 in, 1 out]
            n365 = while {
              tunnel: w718 -> [w735]
              tunnel: w719 -> [w734]
              tunnel: w726 -> [w740]
              tunnel: w726 -> [w739]
              stop <- w741 stop-if-true
              n366 = call <vilib>:"WPI_CANTalonSRX_GetStatus.vi"("CAN Talon SRX Ref"=w735) -> ("Talon SRX Status"=w737:T12)  [unwired: 8 in, 2 out]
              n367 = call <vilib>:"WPI_CANTalonSRX_GetStatus.vi"("CAN Talon SRX Ref"=w734) -> ("Talon SRX Status"=w736:T12)  [unwired: 8 in, 2 out]
              n368 = Wait (ms)(milliseconds to wait=u32 20) -> ()  [unwired: 1 out]
              n369 = Unbundle By Name(w737) -> ("Encoder Position"=w733:dbl)
              n370 = Unbundle By Name(w736) -> ("Encoder Position"=w731:dbl)
              n371 = Negate(x=w733) -> (-x=w732:dbl)
              n372 = Negate(x=w731) -> (-x=w730:dbl)
              n373 = Less Or Equal?(x=w732, y=w740) -> (x <= y?=w743:bool)
              n374 = Less Or Equal?(x=w730, y=w739) -> (x <= y?=w742:bool)
              n375 = And(x=w743, y=w742) -> (x .and. y?=w741:bool)
            }
          }
          frame "End" {
            w748 = 0.0 ("Left axis value")
            # "The autonomous is finished, the encoders are reset for the last time, and the loop stops, ending Autonomous."
            n376 = Unbundle By Name(w750) -> ("DriveRef"=w749:T1)
            n377 = call "Custom Tank.vi"("RobotDriveDevRef 2"=w749, "Left axis value"=w748, "Right axis value"=w748) -> ("Middle Left Motor"=w745:T2, "Middle Right Motor"=w744:T2)  [unwired: 8 in, 3 out]
            n378 = call <vilib>:"WPI_CANTalonSRX_SetSensorPosition.vi"("New Sensor Position"=0.0, "CAN Talon SRX Ref"=w745) -> ()  [unwired: 8 in, 2 out]
            n379 = call <vilib>:"WPI_CANTalonSRX_SetSensorPosition.vi"("New Sensor Position"=0.0, "CAN Talon SRX Ref"=w744) -> ()  [unwired: 8 in, 2 out]
          }
        }
      }
    }
    frame "Position 4" {
      w756 = 0.0  # Rotation Distance
      w757 = 0.0  # Distance from Starting Point
      w758 = FALSE  # End loop?
      w759 = T10."Start"  # Beginning State
      # "Go through low bar, turn right until vision, shoot, return"
      # "Goes through accross Cat B/Cat D defenses, attempts to shoot high, and moves back."
      n380 = while {
        shift-right: [w767] -> _
        shift-left: w759 -> [w768]
        shift-right: [w765] -> _
        shift-left: w758 -> [w766]
        shift-right: [w763] -> _
        shift-left: w757 -> [w764]
        shift-right: [w761] -> _
        shift-left: w756 -> [w762]
        tunnel: w755 -> [w760]
        stop <- w765 stop-if-true
        n381 = case shown="\"Start\", Default" w768 {
          tunnel: [T10."Shoot" T10."Move Back" T10."End" T10."End"] -> w767
          tunnel: [w784 w818 w831 TRUE] -> w765
          tunnel: w766 -> [w784 w818 w831 _]
          tunnel: [w780 w816 w828 w855] -> w763
          tunnel: w764 -> [_ w816 w828 w855]
          tunnel: w762 -> [w779 w815 w830 w854]
          tunnel: [w779 w815 w830 w854] -> w761
          tunnel: w760 -> [w773 w814 w827 w853]
          frame "Start", Default {
            w771 = 0.8 ("LeftMotorsSpeed")
            # "In order to prevent overshooting on the way back, the smaller distance recorded by\neither encoder would be kept."
            # "Stop the motors and bring the arms up 30 degrees so that they would see the goal better"
            # "Set the motors so the robot moves forward at moderate speed"
            n382 = flat-sequence {
              tunnel: [w785] -> w774
              tunnel: w773 -> [w785]
              frame #0 {
                n383 = call "Zero Dart.vi"() -> ()  [unwired: 10 in, 2 out]
              }
            }
            n384 = Unbundle By Name(w774) -> ("DriveRef"=w772:T1)
            n385 = call "Custom Tank.vi"("RobotDriveDevRef 2"=w772, "Left axis value"=w771, "Right axis value"=w771) -> ("Middle Left Motor"=w770:T2, "Middle Right Motor"=w769:T2)  [unwired: 8 in, 3 out]
            n386 = while {
              tunnel: [w790] -> w777
              tunnel: [w786] -> w776
              tunnel: w774 -> [w794]
              tunnel: [w794] -> w775
              tunnel: w770 -> [w791]
              tunnel: w769 -> [w792]
              stop <- w799 stop-if-true
              # "The motors will continue running until both encoders meet the desired distance"
              n387 = call <vilib>:"WPI_CANTalonSRX_GetStatus.vi"("CAN Talon SRX Ref"=w792) -> ("Talon SRX Status"=w793:T12)  [unwired: 8 in, 2 out]
              n388 = Wait (ms)(milliseconds to wait=u32 20) -> ()  [unwired: 1 out]
              n389 = Unbundle By Name(w793) -> ("Encoder Position"=w787:dbl)
              n390 = call <vilib>:"WPI_CANTalonSRX_GetStatus.vi"("CAN Talon SRX Ref"=w791) -> ("Talon SRX Status"=w788:T12)  [unwired: 8 in, 2 out]
              n391 = Unbundle By Name(w788) -> ("Encoder Position"=w789:dbl)
              n392 = Negate(x=w789) -> (-x=w790:dbl)
              n393 = Negate(x=w787) -> (-x=w786:dbl)
              n394 = call "DistanceToEncoder.vi"(8:TRUE ("Gear Setting"), "Distance (in)"=180.0 ("Distance")) -> ("Encoder Ticks"=w796:dbl)  [unwired: 9 in]
              n395 = Greater Or Equal?(x=w790, y=w796) -> (x >= y?=w801:bool)
              n396 = Greater Or Equal?(x=w786, y=w796) -> (x >= y?=w800:bool)
              n397 = And(x=w801, y=w800) -> (x .and. y?=w799:bool)
            }
            n398 = flat-sequence {
              tunnel: [w808] -> w782
              tunnel: [w807] -> w781
              tunnel: w777 -> [w808]
              tunnel: w776 -> [w807]
              tunnel: w775 -> [w806]
              tunnel: [w804] -> _
              frame #0 {
                w802 = 0.0 ("LeftMotorsSpeed")
                n399 = Unbundle By Name(w806) -> ("DriveRef"=w803:T1)
                n400 = call "Set Angle.vi"("Angle(degrees)"=60.0) -> ()  [unwired: 10 in, 1 out]
                n401 = Wait (ms)(milliseconds to wait=u32 2000) -> ()  [unwired: 1 out]
                n402 = global read "Robot Global Data.vi" "Vision Data"() -> (w805:T11)
                n403 = call "Custom Tank.vi"("RobotDriveDevRef 2"=w803, "Left axis value"=w802, "Right axis value"=w802) -> ()  [unwired: 8 in, 5 out]
                n404 = Unbundle By Name(w805) -> ("Distance"=w804:dbl)
              }
            }
            n405 = Less?(x=w782, y=w781) -> (x < y?=w783:bool)
            n406 = Select(t=w782, s=w783, f=w781) -> (s? t:f=w780:dbl)
          }
          frame "Shoot" {
            w811 = 0.0 ("LeftMotorsSpeed")
            # "If they weren't already, the motors of the drive are stopped."
            # "The robot then aligns itself vertically with the goal (also in pixels), charges up the shooting mechanism, and hopefully scores into the goal without problem"
            # "Shoot the boulder"
            n407 = Unbundle By Name(w814) -> ("DriveRef"=w812:T1)
            n408 = call "Shoot.vi"("Trigger"=TRUE ("Collection Trigger")) -> ()  [unwired: 8 in, 3 out]
            n409 = call "Custom Tank.vi"("RobotDriveDevRef 2"=w812, "Left axis value"=w811, "Right axis value"=w811) -> ()  [unwired: 8 in, 5 out]
          }
          frame "Move Back" {
            w825 = -0.75 ("LeftMotorsSpeed")
            # "The robot would then use the previously recorded distance to  move back through the defense in order to get the next boulder as quickly as possible once Teleop starts."
            n410 = Unbundle By Name(w827) -> ("DriveRef"=w826:T1)
            n411 = call "Custom Tank.vi"("RobotDriveDevRef 2"=w826, "Left axis value"=w825, "Right axis value"=w825) -> ("Middle Left Motor"=w822:T2, "Middle Right Motor"=w821:T2)  [unwired: 8 in, 3 out]
            n412 = Negate(x=w828) -> (-x=w829:dbl)
            n413 = call <vilib>:"WPI_CANTalonSRX_SetSensorPosition.vi"("New Sensor Position"=0.0, "CAN Talon SRX Ref"=w822) -> ("CAN Talon SRX Ref"=w820:T2)  [unwired: 8 in, 1 out]
            n414 = call <vilib>:"WPI_CANTalonSRX_SetSensorPosition.vi"("New Sensor Position"=0.0, "CAN Talon SRX Ref"=w821) -> ("CAN Talon SRX Ref"=w819:T2)  [unwired: 8 in, 1 out]
            n415 = while {
              tunnel: w820 -> [w839]
              tunnel: w819 -> [w837]
              tunnel: w829 -> [w843]
              tunnel: w829 -> [w842]
              stop <- w844 stop-if-true
              n416 = call <vilib>:"WPI_CANTalonSRX_GetStatus.vi"("CAN Talon SRX Ref"=w839) -> ("Talon SRX Status"=w840:T12)  [unwired: 8 in, 2 out]
              n417 = call <vilib>:"WPI_CANTalonSRX_GetStatus.vi"("CAN Talon SRX Ref"=w837) -> ("Talon SRX Status"=w838:T12)  [unwired: 8 in, 2 out]
              n418 = Wait (ms)(milliseconds to wait=u32 20) -> ()  [unwired: 1 out]
              n419 = Unbundle By Name(w840) -> ("Encoder Position"=w833:dbl)
              n420 = Unbundle By Name(w838) -> ("Encoder Position"=w834:dbl)
              n421 = Negate(x=w833) -> (-x=w836:dbl)
              n422 = Negate(x=w834) -> (-x=w835:dbl)
              n423 = Less Or Equal?(x=w836, y=w843) -> (x <= y?=w846:bool)
              n424 = Less Or Equal?(x=w835, y=w842) -> (x <= y?=w845:bool)
              n425 = And(x=w846, y=w845) -> (x .and. y?=w844:bool)
            }
          }
          frame "End" {
            w852 = 0.0 ("Left axis value")
            # "The autonomous is finished, the encoders are reset for the last time, and the loop stops, ending Autonomous."
            n426 = Unbundle By Name(w853) -> ("DriveRef"=w849:T1)
            n427 = call "Custom Tank.vi"("RobotDriveDevRef 2"=w849, "Left axis value"=w852, "Right axis value"=w852) -> ("Middle Left Motor"=w848:T2, "Middle Right Motor"=w847:T2)  [unwired: 8 in, 3 out]
            n428 = call <vilib>:"WPI_CANTalonSRX_SetSensorPosition.vi"("New Sensor Position"=0.0, "CAN Talon SRX Ref"=w848) -> ()  [unwired: 8 in, 2 out]
            n429 = call <vilib>:"WPI_CANTalonSRX_SetSensorPosition.vi"("New Sensor Position"=0.0, "CAN Talon SRX Ref"=w847) -> ()  [unwired: 8 in, 2 out]
          }
        }
      }
    }
    frame "Position 5" {
      w861 = 0.0  # Rotation Distance
      w860 = 0.0  # Distance from Starting Point
      w862 = FALSE  # End loop?
      w863 = T10."Start"  # Beginning State
      # "Go through low bar, turn left until vision, shoot, return"
      # "Goes through accross Cat B/Cat D defenses, turns left until the goal is found, attempts to shoot high, and moves back."
      n430 = while {
        shift-right: [w872] -> _
        shift-left: w863 -> [w873]
        shift-right: [w870] -> _
        shift-left: w862 -> [w871]
        shift-right: [w868] -> _
        shift-left: w860 -> [w869]
        shift-right: [w866] -> _
        shift-left: w861 -> [w867]
        tunnel: w859 -> [w865]
        tunnel: w858 -> [w864]
        stop <- w870 stop-if-true
        n431 = case shown="\"Start\", Default" w873 {
          tunnel: [w892 T10."Shoot" T10."Shoot" T10."Turn Back" T10."Move Back" T10."End" T10."End"] -> w872
          tunnel: [w891 w934 w977 w1043 w1057 w1085 TRUE] -> w870
          tunnel: w871 -> [w891 w934 w977 w1043 w1057 w1085 _]
          tunnel: [w885 w933 w976 w1041 w1056 w1082 w1109] -> w868
          tunnel: w869 -> [_ w933 w976 w1041 w1056 w1082 w1109]
          tunnel: w867 -> [w884 _ _ w1040 w1054 w1084 w1108]
          tunnel: [w884 w928 w973 w1040 w1054 w1084 w1108] -> w866
          tunnel: w865 -> [w883 _ _ _ _ _ _]
          tunnel: w864 -> [w878 w926 w968 w1039 w1053 w1081 w1107]
          frame "Start", Default {
            w876 = 0.8 ("LeftMotorsSpeed")
            # "In order to prevent overshooting on the way back, the smaller distance recorded by\neither encoder would be kept."
            # "Stop the motors and bring the arms up 30 degrees so that they would see the goal better"
            # "Set the motors so the robot moves forward at moderate speed"
            # "Changes state depending on whether vision is needed (should be needed at least 99% of the time)"
            n432 = flat-sequence {
              tunnel: w878 -> [w893]
              tunnel: [w893] -> w879
              frame #0 {
                n433 = call "Zero Dart.vi"() -> ()  [unwired: 10 in, 2 out]
              }
            }
            n434 = Unbundle By Name(w879) -> ("DriveRef"=w877:T1)
            n435 = Select(t=T10."Turn (Vision)", s=w883, f=T10."Turn (No Vision)") -> (s? t:f=w892:T10)
            n436 = call "Custom Tank.vi"("RobotDriveDevRef 2"=w877, "Left axis value"=w876, "Right axis value"=w876) -> ("Middle Left Motor"=w875:T2, "Middle Right Motor"=w874:T2)  [unwired: 8 in, 3 out]
            n437 = while {
              tunnel: [w895] -> w881
              tunnel: [w897] -> w882
              tunnel: w879 -> [w903]
              tunnel: [w903] -> w880
              tunnel: w875 -> [w900]
              tunnel: w874 -> [w898]
              stop <- w907 stop-if-true
              # "The motors will continue running until both encoders meet the desired distance"
              n438 = call <vilib>:"WPI_CANTalonSRX_GetStatus.vi"("CAN Talon SRX Ref"=w900) -> ("Talon SRX Status"=w901:T12)  [unwired: 8 in, 2 out]
              n439 = call <vilib>:"WPI_CANTalonSRX_GetStatus.vi"("CAN Talon SRX Ref"=w898) -> ("Talon SRX Status"=w899:T12)  [unwired: 8 in, 2 out]
              n440 = Wait (ms)(milliseconds to wait=u32 20) -> ()  [unwired: 1 out]
              n441 = Unbundle By Name(w901) -> ("Encoder Position"=w894:dbl)
              n442 = Unbundle By Name(w899) -> ("Encoder Position"=w896:dbl)
              n443 = Negate(x=w894) -> (-x=w895:dbl)
              n444 = Negate(x=w896) -> (-x=w897:dbl)
              n445 = call "DistanceToEncoder.vi"(8:TRUE ("Gear Setting"), "Distance (in)"=180.0 ("Distance")) -> ("Encoder Ticks"=w904:dbl)  [unwired: 9 in]
              n446 = Greater Or Equal?(x=w895, y=w904) -> (x >= y?=w909:bool)
              n447 = Greater Or Equal?(x=w897, y=w904) -> (x >= y?=w908:bool)
              n448 = And(x=w909, y=w908) -> (x .and. y?=w907:bool)
            }
            n449 = flat-sequence {
              tunnel: [w913] -> w887
              tunnel: [w914] -> w886
              tunnel: w882 -> [w914]
              tunnel: w881 -> [w913]
              tunnel: w880 -> [w912]
              frame #0 {
                w911 = 0.0 ("LeftMotorsSpeed")
                # "Bring the arms up to a certain angle in order to see the goal later"
                n450 = Unbundle By Name(w912) -> ("DriveRef"=w910:T1)
                n451 = call "Set Angle.vi"("Angle(degrees)"=60.0) -> ()  [unwired: 10 in, 1 out]
                n452 = Wait (ms)(milliseconds to wait=u32 2000) -> ()  [unwired: 1 out]
                n453 = call "Custom Tank.vi"("RobotDriveDevRef 2"=w910, "Left axis value"=w911, "Right axis value"=w911) -> ()  [unwired: 8 in, 5 out]
              }
            }
            n454 = Less?(x=w887, y=w886) -> (x < y?=w888:bool)
            n455 = Select(t=w887, s=w888, f=w886) -> (s? t:f=w885:dbl)
          }
          frame "Turn (No Vision)" {
            # "It is best not to use this code EVER!"
            # "Turn until certain encoder values are reached"
            n456 = Unbundle By Name(w926) -> ("DriveRef"=w925:T1)
            n457 = global read "Robot Global Data.vi" "Vision Data"() -> (w927:T11)
            n458 = call "Custom Tank.vi"("RobotDriveDevRef 2"=w925, "Left axis value"=-0.75 ("LeftMotorsSpeed"), "Right axis value"=0.75 ("RightMotorsSpeed")) -> ("Middle Left Motor"=w921:T2, "Middle Right Motor"=w919:T2)  [unwired: 8 in, 3 out]
            n459 = Unbundle By Name(w927) -> ()  [unwired: 1 out]
            n460 = call <vilib>:"WPI_CANTalonSRX_SetSensorPosition.vi"("New Sensor Position"=0.0, "CAN Talon SRX Ref"=w921) -> ("CAN Talon SRX Ref"=w918:T2)  [unwired: 8 in, 1 out]
            n461 = call <vilib>:"WPI_CANTalonSRX_SetSensorPosition.vi"("New Sensor Position"=0.0, "CAN Talon SRX Ref"=w919) -> ("CAN Talon SRX Ref"=w917:T2)  [unwired: 8 in, 1 out]
            n462 = while {
              tunnel: w917 -> [w941]
              tunnel: w918 -> [w940]
              tunnel: [w936] -> w930
              tunnel: [w939] -> w932
              stop <- w945 stop-if-true
              # "Replace 0s with actual values"
              n463 = call <vilib>:"WPI_CANTalonSRX_GetStatus.vi"("CAN Talon SRX Ref"=w940) -> ("Talon SRX Status"=w943:T12)  [unwired: 8 in, 2 out]
              n464 = call <vilib>:"WPI_CANTalonSRX_GetStatus.vi"("CAN Talon SRX Ref"=w941) -> ("Talon SRX Status"=w942:T12)  [unwired: 8 in, 2 out]
              n465 = Wait (ms)(milliseconds to wait=u32 20) -> ()  [unwired: 1 out]
              n466 = Unbundle By Name(w942) -> ("Encoder Position"=w937:dbl)
              n467 = Unbundle By Name(w943) -> ("Encoder Position"=w938:dbl)
              n468 = Negate(x=w938) -> (-x=w939:dbl)
              n469 = Negate(x=w937) -> (-x=w936:dbl)
              n470 = Greater Or Equal?(x=w936, y=0.0) -> (x >= y?=w948:bool)
              n471 = Less Or Equal?(x=w939, y=-0.0) -> (x <= y?=w947:bool)
              n472 = And(x=w948, y=w947) -> (x .and. y?=w945:bool)
            }
            n473 = Negate(x=w932) -> (-x=w929:dbl)
            n474 = Less?(x=w930, y=w929) -> (x < y?=w931:bool)
            n475 = Select(t=w930, s=w931, f=w929) -> (s? t:f=w928:dbl)
          }
          frame "Turn (Vision)" {
            # "Once again the smaller rotation distance of the two encoders\nare recorded, although one of them is reversed since it was going\nin reverse."
            # "Both motors will stop and the robot checks if the goal is still centered within the range after half a second."
            # "This turn goes on until the x-value of the center of the goal in pixels\nmatches the average x-value between the two (not displayed) cameras."
            # "Since the goal is towards the left, the robot will start turning in place"
            n476 = Unbundle By Name(w968) -> ("DriveRef"=w958:T1)
            n477 = call "Custom Tank.vi"("RobotDriveDevRef 2"=w958, "Left axis value"=-0.75 ("LeftMotorsSpeed"), "Right axis value"=0.75 ("RightMotorsSpeed")) -> ("Middle Left Motor"=w953:T2, "Middle Right Motor"=w952:T2)  [unwired: 8 in, 3 out]
            n478 = call <vilib>:"WPI_CANTalonSRX_SetSensorPosition.vi"("New Sensor Position"=0.0, "CAN Talon SRX Ref"=w953) -> ("CAN Talon SRX Ref"=w951:T2)  [unwired: 8 in, 1 out]
            n479 = call <vilib>:"WPI_CANTalonSRX_SetSensorPosition.vi"("New Sensor Position"=0.0, "CAN Talon SRX Ref"=w952) -> ("CAN Talon SRX Ref"=w950:T2)  [unwired: 8 in, 1 out]
            n480 = while {
              tunnel: w951 -> [w1011]
              tunnel: w950 -> [w1010]
              tunnel: [w1008] -> w969
              tunnel: [w1006] -> w970
              tunnel: w968 -> [w1014]
              tunnel: [w1014] -> w967
              stop <- w1020 stop-if-true
              n481 = call <vilib>:"WPI_CANTalonSRX_GetStatus.vi"("CAN Talon SRX Ref"=w1011) -> ("Talon SRX Status"=w1013:T12)  [unwired: 8 in, 2 out]
              n482 = call <vilib>:"WPI_CANTalonSRX_GetStatus.vi"("CAN Talon SRX Ref"=w1010) -> ("Talon SRX Status"=w1012:T12)  [unwired: 8 in, 2 out]
              n483 = Wait (ms)(milliseconds to wait=u32 20) -> ()  [unwired: 1 out]
              n484 = Unbundle By Name(w1013) -> ("Encoder Position"=w1009:dbl)
              n485 = Unbundle By Name(w1012) -> ("Encoder Position"=w1007:dbl)
              n486 = global read "Robot Global Data.vi" "Vision Data"() -> (w1019:T11)
              n487 = Negate(x=w1007) -> (-x=w1006:dbl)
              n488 = Unbundle By Name(w1019) -> ("x"=w1018:dbl)
              n489 = In Range and Coerce(upper limit=410.0, x=w1018, lower limit=390.0) -> (In Range?=w1020:bool)  [unwired: 1 out]
              n490 = Negate(x=w1009) -> (-x=w1008:dbl)
            }
            n491 = flat-sequence {
              tunnel: [w1024] -> w972
              tunnel: [w1025] -> w971
              tunnel: w970 -> [w1025]
              tunnel: w969 -> [w1024]
              tunnel: w967 -> [w1023]
              tunnel: [w1023] -> w966
              tunnel: w972 -> [w1030]
              tunnel: w971 -> [w1029]
              tunnel: w966 -> [w1031]
              tunnel: [w1031] -> w965
              tunnel: [w1030] -> w964
              tunnel: [w1029] -> w963
              tunnel: [w1028] -> w960
              tunnel: [w1027] -> w959
              frame #0 {
                w1021 = 0.0 ("LeftMotorsSpeed")
                n492 = Unbundle By Name(w1023) -> ("DriveRef"=w1022:T1)
                n493 = Wait (ms)(milliseconds to wait=u32 500) -> ()  [unwired: 1 out]
                n494 = call "Custom Tank.vi"("RobotDriveDevRef 2"=w1022, "Left axis value"=w1021, "Right axis value"=w1021) -> ()  [unwired: 8 in, 5 out]
              }
              frame #1 {
                n495 = global read "Robot Global Data.vi" "Vision Data"() -> (w1035:T11)
                n496 = Unbundle By Name(w1035) -> ("x"=w1034:dbl, "Distance"=w1027:dbl)
                n497 = In Range and Coerce(upper limit=410.0, x=w1034, lower limit=390.0) -> (In Range?=w1028:bool)  [unwired: 1 out]
              }
            }
            n498 = case shown="False" w960 {
              tunnel: [w986 w1005] -> w961
              tunnel: w963 -> [_ w1005]
              tunnel: w964 -> [_ w1004]
              tunnel: [w987 w1004] -> w962
              tunnel: w965 -> [w985 _]
              tunnel: [w984 w1003] -> _
              tunnel: w959 -> [_ w1003]
              frame False {
                # "If it isn't within range then the robot will turn in place in the other direction at a slower pace until the desired pixel range is met"
                n499 = Unbundle By Name(w985) -> ("DriveRef"=w983:T1)
                n500 = call "Custom Tank.vi"("RobotDriveDevRef 2"=w983, "Left axis value"=0.4 ("LeftMotorsSpeed"), "Right axis value"=-0.4 ("RightMotorsSpeed")) -> ("Middle Left Motor"=w980:T2, "Middle Right Motor"=w979:T2)  [unwired: 8 in, 3 out]
                n501 = while {
                  tunnel: [w990] -> w987
                  tunnel: [w988] -> w986
                  tunnel: [w996] -> w984
                  tunnel: w980 -> [w993]
                  tunnel: w979 -> [w992]
                  stop <- w1002 stop-if-true
                  n502 = call <vilib>:"WPI_CANTalonSRX_GetStatus.vi"("CAN Talon SRX Ref"=w993) -> ("Talon SRX Status"=w995:T12)  [unwired: 8 in, 2 out]
                  n503 = call <vilib>:"WPI_CANTalonSRX_GetStatus.vi"("CAN Talon SRX Ref"=w992) -> ("Talon SRX Status"=w994:T12)  [unwired: 8 in, 2 out]
                  n504 = Wait (ms)(milliseconds to wait=u32 20) -> ()  [unwired: 1 out]
                  n505 = Unbundle By Name(w995) -> ("Encoder Position"=w991:dbl)
                  n506 = Unbundle By Name(w994) -> ("Encoder Position"=w989:dbl)
                  n507 = global read "Robot Global Data.vi" "Vision Data"() -> (w1001:T11)
                  n508 = Unbundle By Name(w1001) -> ("x"=w1000:dbl, "Distance"=w996:dbl)
                  n509 = Negate(x=w989) -> (-x=w988:dbl)
                  n510 = In Range and Coerce(upper limit=405.0, x=w1000, lower limit=395.0) -> (In Range?=w1002:bool)  [unwired: 1 out]
                  n511 = Negate(x=w991) -> (-x=w990:dbl)
                }
              }
              frame True {
                # "If it is within range, then the robot moves on to the shooting state"
              }
            }
            n512 = Negate(x=w962) -> (-x=w974:dbl)
            n513 = Less?(x=w961, y=w974) -> (x < y?=w975:bool)
            n514 = Select(t=w961, s=w975, f=w974) -> (s? t:f=w973:dbl)
          }
          frame "Shoot" {
            w1036 = 0.0 ("LeftMotorsSpeed")
            # "If they weren't already, the motors of the drive are stopped."
            # "The robot then aligns itself vertically with the goal (also in pixels), charges up the shooting mechanism, and hopefully scores into the goal without problem"
            n515 = Unbundle By Name(w1039) -> ("DriveRef"=w1037:T1)
            n516 = call "Shoot.vi"("Trigger"=TRUE ("Collection Trigger")) -> ()  [unwired: 8 in, 3 out]
            n517 = call "Custom Tank.vi"("RobotDriveDevRef 2"=w1037, "Left axis value"=w1036, "Right axis value"=w1036) -> ()  [unwired: 8 in, 5 out]
          }
          frame "Turn Back" {
            # "The robot would then use the previously recorded value of rotation to align itself perpendicularly to the defense it came through"
            n518 = Unbundle By Name(w1053) -> ("DriveRef"=w1052:T1)
            n519 = Negate(x=w1054) -> (-x=w1055:dbl)
            n520 = call "Custom Tank.vi"("RobotDriveDevRef 2"=w1052, "Left axis value"=0.75 ("LeftMotorsSpeed"), "Right axis value"=-0.75 ("RightMotorsSpeed")) -> ("Middle Left Motor"=w1047:T2, "Middle Right Motor"=w1046:T2)  [unwired: 8 in, 3 out]
            n521 = call <vilib>:"WPI_CANTalonSRX_SetSensorPosition.vi"("New Sensor Position"=0.0, "CAN Talon SRX Ref"=w1047) -> ("CAN Talon SRX Ref"=w1044:T2)  [unwired: 8 in, 1 out]
            n522 = call <vilib>:"WPI_CANTalonSRX_SetSensorPosition.vi"("New Sensor Position"=0.0, "CAN Talon SRX Ref"=w1046) -> ("CAN Talon SRX Ref"=w1045:T2)  [unwired: 8 in, 1 out]
            n523 = while {
              tunnel: w1045 -> [w1064]
              tunnel: w1044 -> [w1063]
              tunnel: w1054 -> [w1069]
              tunnel: w1055 -> [w1068]
              stop <- w1070 stop-if-true
              n524 = call <vilib>:"WPI_CANTalonSRX_GetStatus.vi"("CAN Talon SRX Ref"=w1063) -> ("Talon SRX Status"=w1066:T12)  [unwired: 8 in, 2 out]
              n525 = call <vilib>:"WPI_CANTalonSRX_GetStatus.vi"("CAN Talon SRX Ref"=w1064) -> ("Talon SRX Status"=w1065:T12)  [unwired: 8 in, 2 out]
              n526 = Wait (ms)(milliseconds to wait=u32 20) -> ()  [unwired: 1 out]
              n527 = Unbundle By Name(w1066) -> ("Encoder Position"=w1059:dbl)
              n528 = Unbundle By Name(w1065) -> ("Encoder Position"=w1061:dbl)
              n529 = Negate(x=w1059) -> (-x=w1060:dbl)
              n530 = Negate(x=w1061) -> (-x=w1062:dbl)
              n531 = Less Or Equal?(x=w1062, y=w1068) -> (x <= y?=w1072:bool)
              n532 = Greater Or Equal?(x=w1060, y=w1069) -> (x >= y?=w1071:bool)
              n533 = And(x=w1072, y=w1071) -> (x .and. y?=w1070:bool)
            }
          }
          frame "Move Back" {
            w1079 = -0.75 ("LeftMotorsSpeed")
            # "The robot would then use the previously recorded distance to  move back through the defense in order to get the next boulder as quickly as possible once Teleop starts."
            n534 = Unbundle By Name(w1081) -> ("DriveRef"=w1080:T1)
            n535 = call "Custom Tank.vi"("RobotDriveDevRef 2"=w1080, "Left axis value"=w1079, "Right axis value"=w1079) -> ("Middle Left Motor"=w1077:T2, "Middle Right Motor"=w1075:T2)  [unwired: 8 in, 3 out]
            n536 = Negate(x=w1082) -> (-x=w1083:dbl)
            n537 = call <vilib>:"WPI_CANTalonSRX_SetSensorPosition.vi"("New Sensor Position"=0.0, "CAN Talon SRX Ref"=w1077) -> ("CAN Talon SRX Ref"=w1074:T2)  [unwired: 8 in, 1 out]
            n538 = call <vilib>:"WPI_CANTalonSRX_SetSensorPosition.vi"("New Sensor Position"=0.0, "CAN Talon SRX Ref"=w1075) -> ("CAN Talon SRX Ref"=w1073:T2)  [unwired: 8 in, 1 out]
            n539 = while {
              tunnel: w1074 -> [w1092]
              tunnel: w1073 -> [w1091]
              tunnel: w1083 -> [w1097]
              tunnel: w1083 -> [w1096]
              stop <- w1098 stop-if-true
              # "Move back to start"
              n540 = call <vilib>:"WPI_CANTalonSRX_GetStatus.vi"("CAN Talon SRX Ref"=w1092) -> ("Talon SRX Status"=w1094:T12)  [unwired: 8 in, 2 out]
              n541 = call <vilib>:"WPI_CANTalonSRX_GetStatus.vi"("CAN Talon SRX Ref"=w1091) -> ("Talon SRX Status"=w1093:T12)  [unwired: 8 in, 2 out]
              n542 = Wait (ms)(milliseconds to wait=u32 20) -> ()  [unwired: 1 out]
              n543 = Unbundle By Name(w1094) -> ("Encoder Position"=w1089:dbl)
              n544 = Unbundle By Name(w1093) -> ("Encoder Position"=w1087:dbl)
              n545 = Negate(x=w1089) -> (-x=w1090:dbl)
              n546 = Negate(x=w1087) -> (-x=w1088:dbl)
              n547 = Less Or Equal?(x=w1090, y=w1097) -> (x <= y?=w1100:bool)
              n548 = Less Or Equal?(x=w1088, y=w1096) -> (x <= y?=w1099:bool)
              n549 = And(x=w1100, y=w1099) -> (x .and. y?=w1098:bool)
            }
          }
          frame "End" {
            w1105 = 0.0 ("Left axis value")
            # "The autonomous is finished, the encoders are reset for the last time, and the loop stops, ending Autonomous."
            n550 = Unbundle By Name(w1107) -> ("DriveRef"=w1106:T1)
            n551 = call "Custom Tank.vi"("RobotDriveDevRef 2"=w1106, "Left axis value"=w1105, "Right axis value"=w1105) -> ("Middle Left Motor"=w1102:T2, "Middle Right Motor"=w1101:T2)  [unwired: 8 in, 3 out]
            n552 = call <vilib>:"WPI_CANTalonSRX_SetSensorPosition.vi"("New Sensor Position"=0.0, "CAN Talon SRX Ref"=w1102) -> ()  [unwired: 8 in, 2 out]
            n553 = call <vilib>:"WPI_CANTalonSRX_SetSensorPosition.vi"("New Sensor Position"=0.0, "CAN Talon SRX Ref"=w1101) -> ()  [unwired: 8 in, 2 out]
          }
        }
      }
    }
    frame "Move Forward through Defense", Default {
      w1117 = 0.8 ("LeftMotorsSpeed")
      # "Set the motors so the robot moves forward at moderate speed"
      # "Only moves the robot through the defense"
      n554 = flat-sequence {
        tunnel: w1114 -> [w1118]
        tunnel: w1114 -> [w1119]
        tunnel: [w1119] -> w1113
        tunnel: [w1118] -> w1112
        tunnel: [w1125] -> w1115
        tunnel: w1113 -> [w1125]
        tunnel: w1112 -> [w1120]
        tunnel: w1115 -> [w1142]
        frame #0 {
          n555 = call "Zero Dart.vi"() -> ()  [unwired: 10 in, 2 out]
        }
        frame #1 {
          w1122 = 0.8 ("LeftMotorsSpeed")
          n556 = Unbundle By Name(w1120) -> ("DriveRef"=w1121:T1)
          n557 = call "Custom Tank.vi"("RobotDriveDevRef 2"=w1121, "Left axis value"=w1122, "Right axis value"=w1122) -> ("Middle Left Motor"=w1123:T2, "Middle Right Motor"=w1124:T2)  [unwired: 8 in, 3 out]
          n558 = while {
            tunnel: [w1128] -> _
            tunnel: [w1126] -> _
            tunnel: [w1135] -> _
            tunnel: w1120 -> [w1135]
            tunnel: w1123 -> [w1131]
            tunnel: w1124 -> [w1130]
            stop <- w1139 stop-if-true
            # "The motors will continue running until both encoders meet the desired distance"
            n559 = call <vilib>:"WPI_CANTalonSRX_GetStatus.vi"("CAN Talon SRX Ref"=w1131) -> ("Talon SRX Status"=w1133:T12)  [unwired: 8 in, 2 out]
            n560 = call <vilib>:"WPI_CANTalonSRX_GetStatus.vi"("CAN Talon SRX Ref"=w1130) -> ("Talon SRX Status"=w1132:T12)  [unwired: 8 in, 2 out]
            n561 = Wait (ms)(milliseconds to wait=u32 20) -> ()  [unwired: 1 out]
            n562 = Unbundle By Name(w1133) -> ("Encoder Position"=w1129:dbl)
            n563 = Unbundle By Name(w1132) -> ("Encoder Position"=w1127:dbl)
            n564 = Negate(x=w1129) -> (-x=w1128:dbl)
            n565 = Negate(x=w1127) -> (-x=w1126:dbl)
            n566 = call "DistanceToEncoder.vi"(8:TRUE ("Gear Setting"), "Distance (in)"=180.0) -> ("Encoder Ticks"=w1137:dbl)  [unwired: 9 in]
            n567 = Greater Or Equal?(x=w1128, y=w1137) -> (x >= y?=w1141:bool)
            n568 = Greater Or Equal?(x=w1126, y=w1137) -> (x >= y?=w1140:bool)
            n569 = And(x=w1141, y=w1140) -> (x .and. y?=w1139:bool)
          }
        }
        frame #2 {
          (unwired) TRUE ("Success?")
          w1147 = 0.0 ("LeftMotorsSpeed")
          n570 = Unbundle By Name(w1142) -> ("DriveRef"=w1148:T1)
          n571 = call "Custom Tank.vi"("RobotDriveDevRef 2"=w1148, "Left axis value"=w1147, "Right axis value"=w1147) -> ("Middle Left Motor"=w1144:T2, "Middle Right Motor"=w1143:T2)  [unwired: 8 in, 3 out]
          n572 = call <vilib>:"WPI_CANTalonSRX_SetSensorPosition.vi"("New Sensor Position"=0.0, "CAN Talon SRX Ref"=w1144) -> ()  [unwired: 8 in, 2 out]
          n573 = call <vilib>:"WPI_CANTalonSRX_SetSensorPosition.vi"("New Sensor Position"=0.0, "CAN Talon SRX Ref"=w1143) -> ()  [unwired: 8 in, 2 out]
        }
      }
      n574 = Unbundle By Name(w1114) -> ("DriveRef"=w1116:T1)
      n575 = call "Custom Tank.vi"("RobotDriveDevRef 2"=w1116, "Left axis value"=w1117, "Right axis value"=w1117) -> ()  [unwired: 8 in, 5 out]
    }
    frame "Turn Until Vision Test" {
      # "Both motors will stop and the robot checks if the goal is still centered within the range after half a second."
      # "This turn goes on until the x-value of the center of the goal in pixels\nmatches the average x-value between the two (not displayed) cameras."
      # "Since the goal is towards the left, the robot will start turning in place"
      # "Turns the robot right until it sees the goal"
      n576 = Unbundle By Name(w1149) -> ("DriveRef"=w1159:T1)
      n577 = call "Custom Tank.vi"("RobotDriveDevRef 2"=w1159, "Left axis value"=0.75 ("LeftMotorsSpeed"), "Right axis value"=-0.75 ("RightMotorsSpeed")) -> ("Middle Left Motor"=w1166:T2, "Middle Right Motor"=w1167:T2)  [unwired: 8 in, 3 out]
      n578 = call <vilib>:"WPI_CANTalonSRX_SetSensorPosition.vi"("New Sensor Position"=0.0, "CAN Talon SRX Ref"=w1166) -> ("CAN Talon SRX Ref"=w1164:T2)  [unwired: 8 in, 1 out]
      n579 = call <vilib>:"WPI_CANTalonSRX_SetSensorPosition.vi"("New Sensor Position"=0.0, "CAN Talon SRX Ref"=w1167) -> ("CAN Talon SRX Ref"=w1165:T2)  [unwired: 8 in, 1 out]
      n580 = while {
        tunnel: w1164 -> [w1204]
        tunnel: w1165 -> [w1205]
        tunnel: [w1200] -> w1151
        tunnel: [w1201] -> w1150
        tunnel: w1149 -> [w1208]
        tunnel: [w1208] -> w1152
        stop <- w1214 stop-if-true
        n581 = call <vilib>:"WPI_CANTalonSRX_GetStatus.vi"("CAN Talon SRX Ref"=w1204) -> ("Talon SRX Status"=w1207:T12)  [unwired: 8 in, 2 out]
        n582 = call <vilib>:"WPI_CANTalonSRX_GetStatus.vi"("CAN Talon SRX Ref"=w1205) -> ("Talon SRX Status"=w1206:T12)  [unwired: 8 in, 2 out]
        n583 = Wait (ms)(milliseconds to wait=u32 20) -> ()  [unwired: 1 out]
        n584 = Unbundle By Name(w1207) -> ("Encoder Position"=w1203:dbl)
        n585 = Unbundle By Name(w1206) -> ("Encoder Position"=w1202:dbl)
        n586 = global read "Robot Global Data.vi" "Vision Data"() -> (w1213:T11)
        n587 = Unbundle By Name(w1213) -> ("x"=w1212:dbl)
        n588 = In Range and Coerce(upper limit=410.0, x=w1212, lower limit=390.0) -> (In Range?=w1214:bool)  [unwired: 1 out]
        n589 = Negate(x=w1203) -> (-x=w1200:dbl)
        n590 = Negate(x=w1202) -> (-x=w1201:dbl)
      }
      n591 = flat-sequence {
        tunnel: [w1218] -> w1170
        tunnel: [w1219] -> w1169
        tunnel: w1150 -> [w1219]
        tunnel: w1151 -> [w1218]
        tunnel: w1152 -> [w1217]
        tunnel: [w1217] -> w1168
        tunnel: w1170 -> [w1224]
        tunnel: w1169 -> [w1223]
        tunnel: w1168 -> [w1225]
        tunnel: [w1225] -> w1153
        tunnel: [w1224] -> w1154
        tunnel: [w1223] -> w1155
        tunnel: [w1222] -> w1156
        tunnel: [w1221] -> w1157
        frame #0 {
          w1215 = 0.0 ("LeftMotorsSpeed")
          n592 = Unbundle By Name(w1217) -> ("DriveRef"=w1216:T1)
          n593 = Wait (ms)(milliseconds to wait=u32 500) -> ()  [unwired: 1 out]
          n594 = call "Custom Tank.vi"("RobotDriveDevRef 2"=w1216, "Left axis value"=w1215, "Right axis value"=w1215) -> ()  [unwired: 8 in, 5 out]
        }
        frame #1 {
          n595 = global read "Robot Global Data.vi" "Vision Data"() -> (w1229:T11)
          n596 = Unbundle By Name(w1229) -> ("x"=w1228:dbl, "Distance"=w1221:dbl)
          n597 = In Range and Coerce(upper limit=410.0, x=w1228, lower limit=390.0) -> (In Range?=w1222:bool)  [unwired: 1 out]
        }
      }
      n598 = case shown="False" w1156 {
        tunnel: [w1179 w1199] -> _
        tunnel: w1155 -> [_ w1199]
        tunnel: w1154 -> [_ w1198]
        tunnel: [w1180 w1198] -> _
        tunnel: w1153 -> [w1178 _]
        tunnel: [w1177 w1197] -> _
        tunnel: w1157 -> [_ w1197]
        tunnel: [TRUE ("End?") TRUE ("End?")] -> w1158
        frame False {
          # "If it isn't within range then the robot will turn in place in the other direction at a slower pace until the desired pixel range is met"
          n599 = Unbundle By Name(w1178) -> ("DriveRef"=w1175:T1)
          n600 = call "Custom Tank.vi"("RobotDriveDevRef 2"=w1175, "Left axis value"=-0.4 ("LeftMotorsSpeed"), "Right axis value"=0.4 ("RightMotorsSpeed")) -> ("Middle Left Motor"=w1172:T2, "Middle Right Motor"=w1171:T2)  [unwired: 8 in, 3 out]
          n601 = while {
            tunnel: [w1183] -> w1180
            tunnel: [w1181] -> w1179
            tunnel: [w1189] -> w1177
            tunnel: w1172 -> [w1186]
            tunnel: w1171 -> [w1185]
            stop <- w1195 stop-if-true
            n602 = call <vilib>:"WPI_CANTalonSRX_GetStatus.vi"("CAN Talon SRX Ref"=w1186) -> ("Talon SRX Status"=w1188:T12)  [unwired: 8 in, 2 out]
            n603 = call <vilib>:"WPI_CANTalonSRX_GetStatus.vi"("CAN Talon SRX Ref"=w1185) -> ("Talon SRX Status"=w1187:T12)  [unwired: 8 in, 2 out]
            n604 = Wait (ms)(milliseconds to wait=u32 20) -> ()  [unwired: 1 out]
            n605 = Unbundle By Name(w1188) -> ("Encoder Position"=w1184:dbl)
            n606 = Unbundle By Name(w1187) -> ("Encoder Position"=w1182:dbl)
            n607 = global read "Robot Global Data.vi" "Vision Data"() -> (w1194:T11)
            n608 = Unbundle By Name(w1194) -> ("x"=w1193:dbl, "Distance"=w1189:dbl)
            n609 = Negate(x=w1182) -> (-x=w1181:dbl)
            n610 = In Range and Coerce(upper limit=405.0, x=w1193, lower limit=395.0) -> (In Range?=w1195:bool)  [unwired: 1 out]
            n611 = Negate(x=w1184) -> (-x=w1183:dbl)
          }
        }
        frame True {
          # "If it is within range, then the robot moves on to the shooting state"
        }
      }
      "End?" <- w1158
    }
    frame "Move Arms Down/Up Test" {
      # "I hope Brian's code works"
      n612 = flat-sequence {
        frame #0 {
          n613 = call "Zero Dart.vi"() -> ()  [unwired: 10 in, 2 out]
        }
        frame #1 {
          n614 = while {
            stop <- "stop?" stop-if-true
            n615 = call "Set Angle.vi"("Angle(degrees)"="Angle(degrees)") -> ()  [unwired: 10 in, 1 out]
          }
        }
      }
    }
  }
